vi "Aerotech Controller Module Assembly (main).vi"() -> ()   [LabVIEW 2011]
uses:
  Control 1.ctl
  C:/Users/Admin/Desktop/Gantry Code Transfer/source/Code Transfer/Aerotech.A3200.dll
  Aerotech.A3200.dll
  <vilib>/Utility/error.llb/whitespace.ctl
  <vilib>/Utility/file.llb/Write To Spreadsheet File (DBL).vi
  <vilib>/Utility/file.llb/Write To Spreadsheet File (string).vi
  <vilib>/Utility/file.llb/Read From Spreadsheet File (DBL).vi
panel:
  in  "Load Stored Vectors":bool
  out "Vertical vector":dbl[](array[numeric])
  out "In Range?":bool
  out "Matched?":bool
  out "Match Score":dbl
  out "Station F":bool[](array[boolean])
  out "Station E":bool[](array[boolean])
  in  "Standard Orientation":bool=TRUE
  in  "Station":string
  in  "Module":string
  in  "AlignmentButton":bool
  out "Station A":bool[](array[boolean])
  out "Station B":bool[](array[boolean])
  in  "Stored Vector to Spreadsheet":bool
  out "Encapsulation Pressure":bool
  out "Station D":bool[](array[boolean])
  out "Station C":bool[](array[boolean])
  in  "Storage and Points":enum32{"Stored Vectors", "Index Points"}(tab)
  out "Stored Vectors":T1[][](array[typedef])
  in  "Index Points":string[][](table)
  out "Lock Increment":bool
  in  "Command Array":dbl[][](array[numeric])
  out "Rotation Offset":dbl
  out "Rotate State":bool
  out "Offset":dbl[](array[numeric])
  out "Joystick state":bool
  out "Play/Pause State":bool
  out "Offset State":bool
  out "step stop":bool
  out "goto next state":bool
  out "Current Position":dbl[](array[numeric])=[0.0, -0.0, -0.0, 5.000003999999996] format="%#.3f"
  out "Gantry Head":bool[](array[boolean])
  out "Needle Pressure State":bool
  out "Limit Tripped":bool
  out "Touching":bool
  out "Wait Time":string
  out "Command log":string="\r>"
  in  "Clear Log":bool
  in  "Stop And reset Sequence":bool
  in  "Information":T2(tab)
  in  "Commands":T3(tab)
  in  "Maintenance Position":bool
  in  "Re-Intialize Stored Vectors":bool
  in  "Only Z?":bool
  out "All Axis Mask":i32
  in  "Home button":bool
  in  "Init button":bool
  in  "Axis Indices":u32[](array[ring])=[0, 2, 3, 4] items=["AXIS 1", "AXIS 2", "AXIS 3", "AXIS 4", "AXIS 5", "AXIS 6", "AXIS 7", "AXIS 8", "AXIS 9", "AXIS 10", "AXIS 11", "AXIS 12", "AXIS 13", "AXIS 14", "AXIS 15", "AXIS 16", "AXIS 17", "AXIS 18", "AXIS 19", "AXIS 20", "AXIS 21", "AXIS 22", "AXIS 23", "AXIS 24", "AXIS 25", "AXIS 26", "AXIS 27", "AXIS 28", "AXIS 29", "AXIS 30", "AXIS 31", "AXIS 32"]
  out "CONTROLLER":refnum<k24>
  in  "Autofocus":bool
  in  "Speed":dbl=20.0
  in  "Index Num":dbl
  in  "Index Move":bool
  in  "Angular Speed (deg/s":dbl=2.0
  in  "Use Stored Point?":bool
  in  "Stored Point #":dbl
  in  "Vector Move":bool
  in  "Relative Motion?":bool
  in  "Position (mm)":dbl[](array[numeric])=[0.0, 0.0, 0.0, 0.0]
  in  "Speed (mm/s)":dbl=20.0
  in  "Enable Joystick":bool
  in  "Use Camera?":bool
  in  "Encapsulation Purge":bool
  in  "Set Needle Pressure":bool
  in  "Set Syringe":bool
  in  "Gantry Head Vacuums":bool[](array[boolean])=[FALSE, FALSE, FALSE, FALSE, FALSE, FALSE, FALSE]
  in  "Run Gantry Head Vacuums":bool
  in  "Station Vacuum Controls":enum32{"A", "B", "C", "D", "E", "F"}(tab)
  in  "A \nVacuums":bool[](array[boolean])=[FALSE, FALSE, FALSE, FALSE]
  in  "Run A Vac.":bool
  in  "B Vacuums":bool[](array[boolean])=[FALSE, FALSE, FALSE, FALSE]
  in  "Run B Vac.":bool
  in  "Run C Vacuums":bool
  in  "C Vacuums":bool[](array[boolean])=[FALSE, FALSE, FALSE, FALSE, FALSE, FALSE, FALSE]
  in  "Run D Vacuums":bool
  in  "D Vacuums":bool[](array[boolean])=[FALSE, FALSE, FALSE, FALSE, FALSE, FALSE, FALSE]
  in  "E Vacuums":bool[](array[boolean])=[FALSE, FALSE, FALSE, FALSE, FALSE, FALSE, FALSE]
  in  "Run E Vacuums":bool
  in  "Run F Vacuums":bool
  in  "F Vacuums":bool[](array[boolean])=[FALSE, FALSE, FALSE, FALSE, FALSE, FALSE, FALSE]
  in  "store to":dbl
  in  "point 3":dbl
  in  "point 2":dbl
  in  "point 1":dbl
  in  "center of circle":bool
  in  "Store to":dbl
  in  "Rotate Vector":bool
  in  "Just 3D?":bool
  in  "Store to #'":dbl
  in  "Vector 2":dbl
  in  "Vector 1":dbl
  in  "Calculate Angle":bool
  in  "Store Unit":dbl
  in  "Unitize button":bool
  in  "Unit Vector?":dbl
  in  "Store to Point":dbl
  in  "Scale Vector":bool
  in  "Vector Location":dbl
  in  "Multiplier":dbl
  in  "Store to Vector Pos.":dbl
  in  "Add Vectors":bool
  in  "Add to Vector":dbl
  in  "Vector Addition":dbl[](array[numeric])=[0.0, 0.0, 0.0, 0.0]
  in  "Offset Position":dbl
  in  "Offset from Stored Vector":bool
  in  "Point 1":dbl
  in  "Point 2":dbl
  in  "Store point":dbl
  in  "Distance 2":bool
  in  "Center 2":bool
  in  "Load Index":bool
  in  "Offset Vector":dbl[](array[numeric])=[0.0, 0.0, 0.0, 0.0]
  in  "Set Offset":bool
  in  "Offset Enabled?":bool
  in  "Set Offset State":bool
  in  "Vector to Store":dbl[](array[numeric])=[0.0, 0.0, 0.0, 0.0]
  in  "Store to #":dbl
  in  "Store Vector":bool
  in  "Use Input Vector":bool
  in  "Pt 1":dbl
  in  "Pt 2":dbl
  in  "Store pt":dbl
  in  "Distance":bool
  in  "Center":bool
  in  "Stored point":dbl
  in  "rotation options":dbl
  in  "angle of rotation":dbl
  in  "Wirebond Template":dbl
  in  "Top/Bottom/Left/Right":dbl
  in  "Type of Wire Bond":dbl
  in  "Scan direction T/B":dbl
  in  "Scan direction R/L":dbl
  in  "Wire Bond Finder":bool
  in  "Store rel match to":dbl
  in  "Fiducial Match":bool
  in  "Min Match Score":dbl=600.0
  in  "Move?":bool
  in  "Type of Pat \nMatch":dbl
  in  "Minimum Match Score":sgl=700.0
  out "Faults":string[](array[string])
  in  "Ack Fault":bool
  out "error out":errorcluster
  in  "Command Table":string[][](table)
  in  "Goto Line":bool
  in  "Goto Line Number":dbl
  in  "Load File":bool
  out "Script Details":string
  out "Current Command number":dbl
  in  "Start-Pause":bool
  in  "Step Button":bool
  in  "Zoomtofit":bool
  out "Image":T4(plugin-control)
  out "Image Out":T4(plugin-control)
  in  "movement abort":bool
  in  "EXIT":bool
  # "USE EXIT VI TO STOP PROGRAM PLEASE!"
  # "Y\n\nX\n\nZ\n\nRot"
  # "Right Chuck (HDI)"
  # "Right Chuck (HDI)"
  # "Pickup Head"
  # "Right Chuck (HDI)"
  # "Left Chuck (Module)"
  # "Left Chuck (Module)"
  # "Radial Pickup Head"
  # "Left Chuck (Module)"
  # "Right bridge hold down"
  # "Right bridge hold down"
  # "Center Vacuum"
  # "Right bridge hold down"
  # "Left bridge hold down"
  # "Left bridge hold down"
  # "Left bridge hold down"
  # "Right Chuck (HDI)"
  # "Right Chuck (HDI)"
  # "Right Chuck (HDI)"
  # "Left Chuck (Module)"
  # "Left Chuck (Module)"
  # "Left Chuck (Module)"
  # "Right bridge hold down"
  # "Right bridge hold down"
  # "Right bridge hold down"
  # "Left bridge hold down"
  # "Left bridge hold down"
  # "Left bridge hold down"
  # "0"
  # "1"
  # "2"
  # "3"
  # "4"
  # "5"
  # "6"
  # "7"
  # "8"
  # "9"
  # "10"
  # "Y\n\nX\n\nZ\n\nRot"
  # "Pickup Head"
  # "Radial Pickup Head"
  # "Center Vacuum"
  # "Right Chuck (HDI)"
  # "Left Chuck (Module)"
  # "Right bridge hold down"
  # "Left bridge hold down"
  # "Right Chuck (HDI)"
  # "Left Chuck (Module)"
  # "Right bridge hold down"
  # "Left bridge hold down"
  # "Right Chuck (HDI)"
  # "Left Chuck (Module)"
  # "Right bridge hold down"
  # "Left bridge hold down"
  # "Right Chuck (HDI)"
  # "Left Chuck (Module)"
  # "Right bridge hold down"
  # "Left bridge hold down"
  # "Right Chuck (HDI)"
  # "Left Chuck (Module)"
  # "Right bridge hold down"
  # "Left bridge hold down"
  # "Right Chuck (HDI)"
  # "Left Chuck (Module)"
  # "Right bridge hold down"
  # "Left bridge hold down"
  # "Lateral 2D"
  # "Lateral 3D"
  # "Type of Pattern Match\n0. Nothing\n1. Sensor Fiducial\n2. TR HDI bond pad \n3. TL -----------------\n4. BL -----------------\n5. Simple Edge Scan"
  # "R/L\n0=right to left\n1=left to right\nT/B \n0=top to bottom\n1=bottom to top"
  # "Wire Bond Pattern Matching"
  # "Top/Bottom/Left/Right Pad\n0. Top       2. Left\n1. Bottom  3. Right"
  # "Type of Wire Bond\n0. ROC\n1. HDI\n2. TBM HDI\n3. TBM TOP\n4. Address Bond"
  # "Template\n0. ROC Pad\n1. HDI Pad\n2. RT TBM HDI Pad\n3. RB TBM HDI Pad\n4. BR TBM HDI Pad\n5. BL TBM HDI Pad\n6. LB TBM HDI Pad\n7. LT TBM HDI Pad\n8. TL TBM HDI Pad\n9. TR TBM HDI Pad\n10. TBM TOP TR\n11. TBM TOP BR\n12. TBM TOP BL\n13. TBM TOP TL\n14. Address Bond Top\n15. Address Bond Bottom"
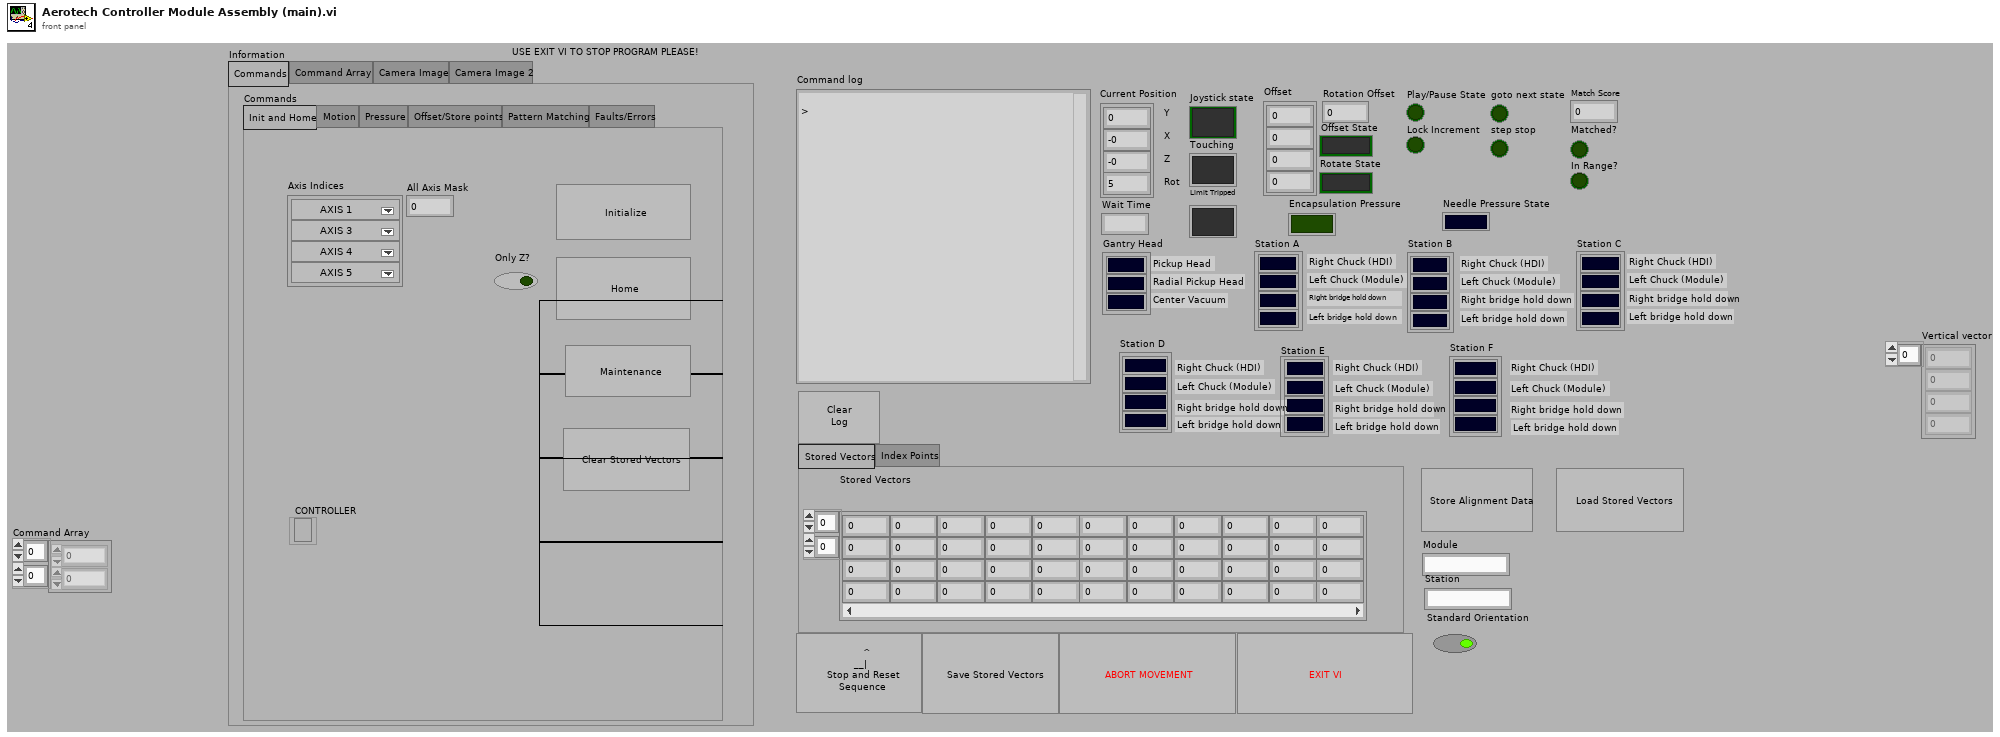
[diagram p1: front panel]
types:
  T1 = typedef "Control 1.ctl" = dbl
  T2 = enum32{"Commands", "Command Array", "Camera Image", "Camera Image 2"}
  T3 = enum32{"Init and Home", "Motion", "Pressure", "Offset/Store points", "Pattern Matching", "Faults/Errors"}
  T4 = typedef "IMAQ Image.ctl" = refnum<image>
  T5 = enum32{"Commands", "Command Array", "Camera Image"}
  T6 = typedef "whitespace.ctl" = u16
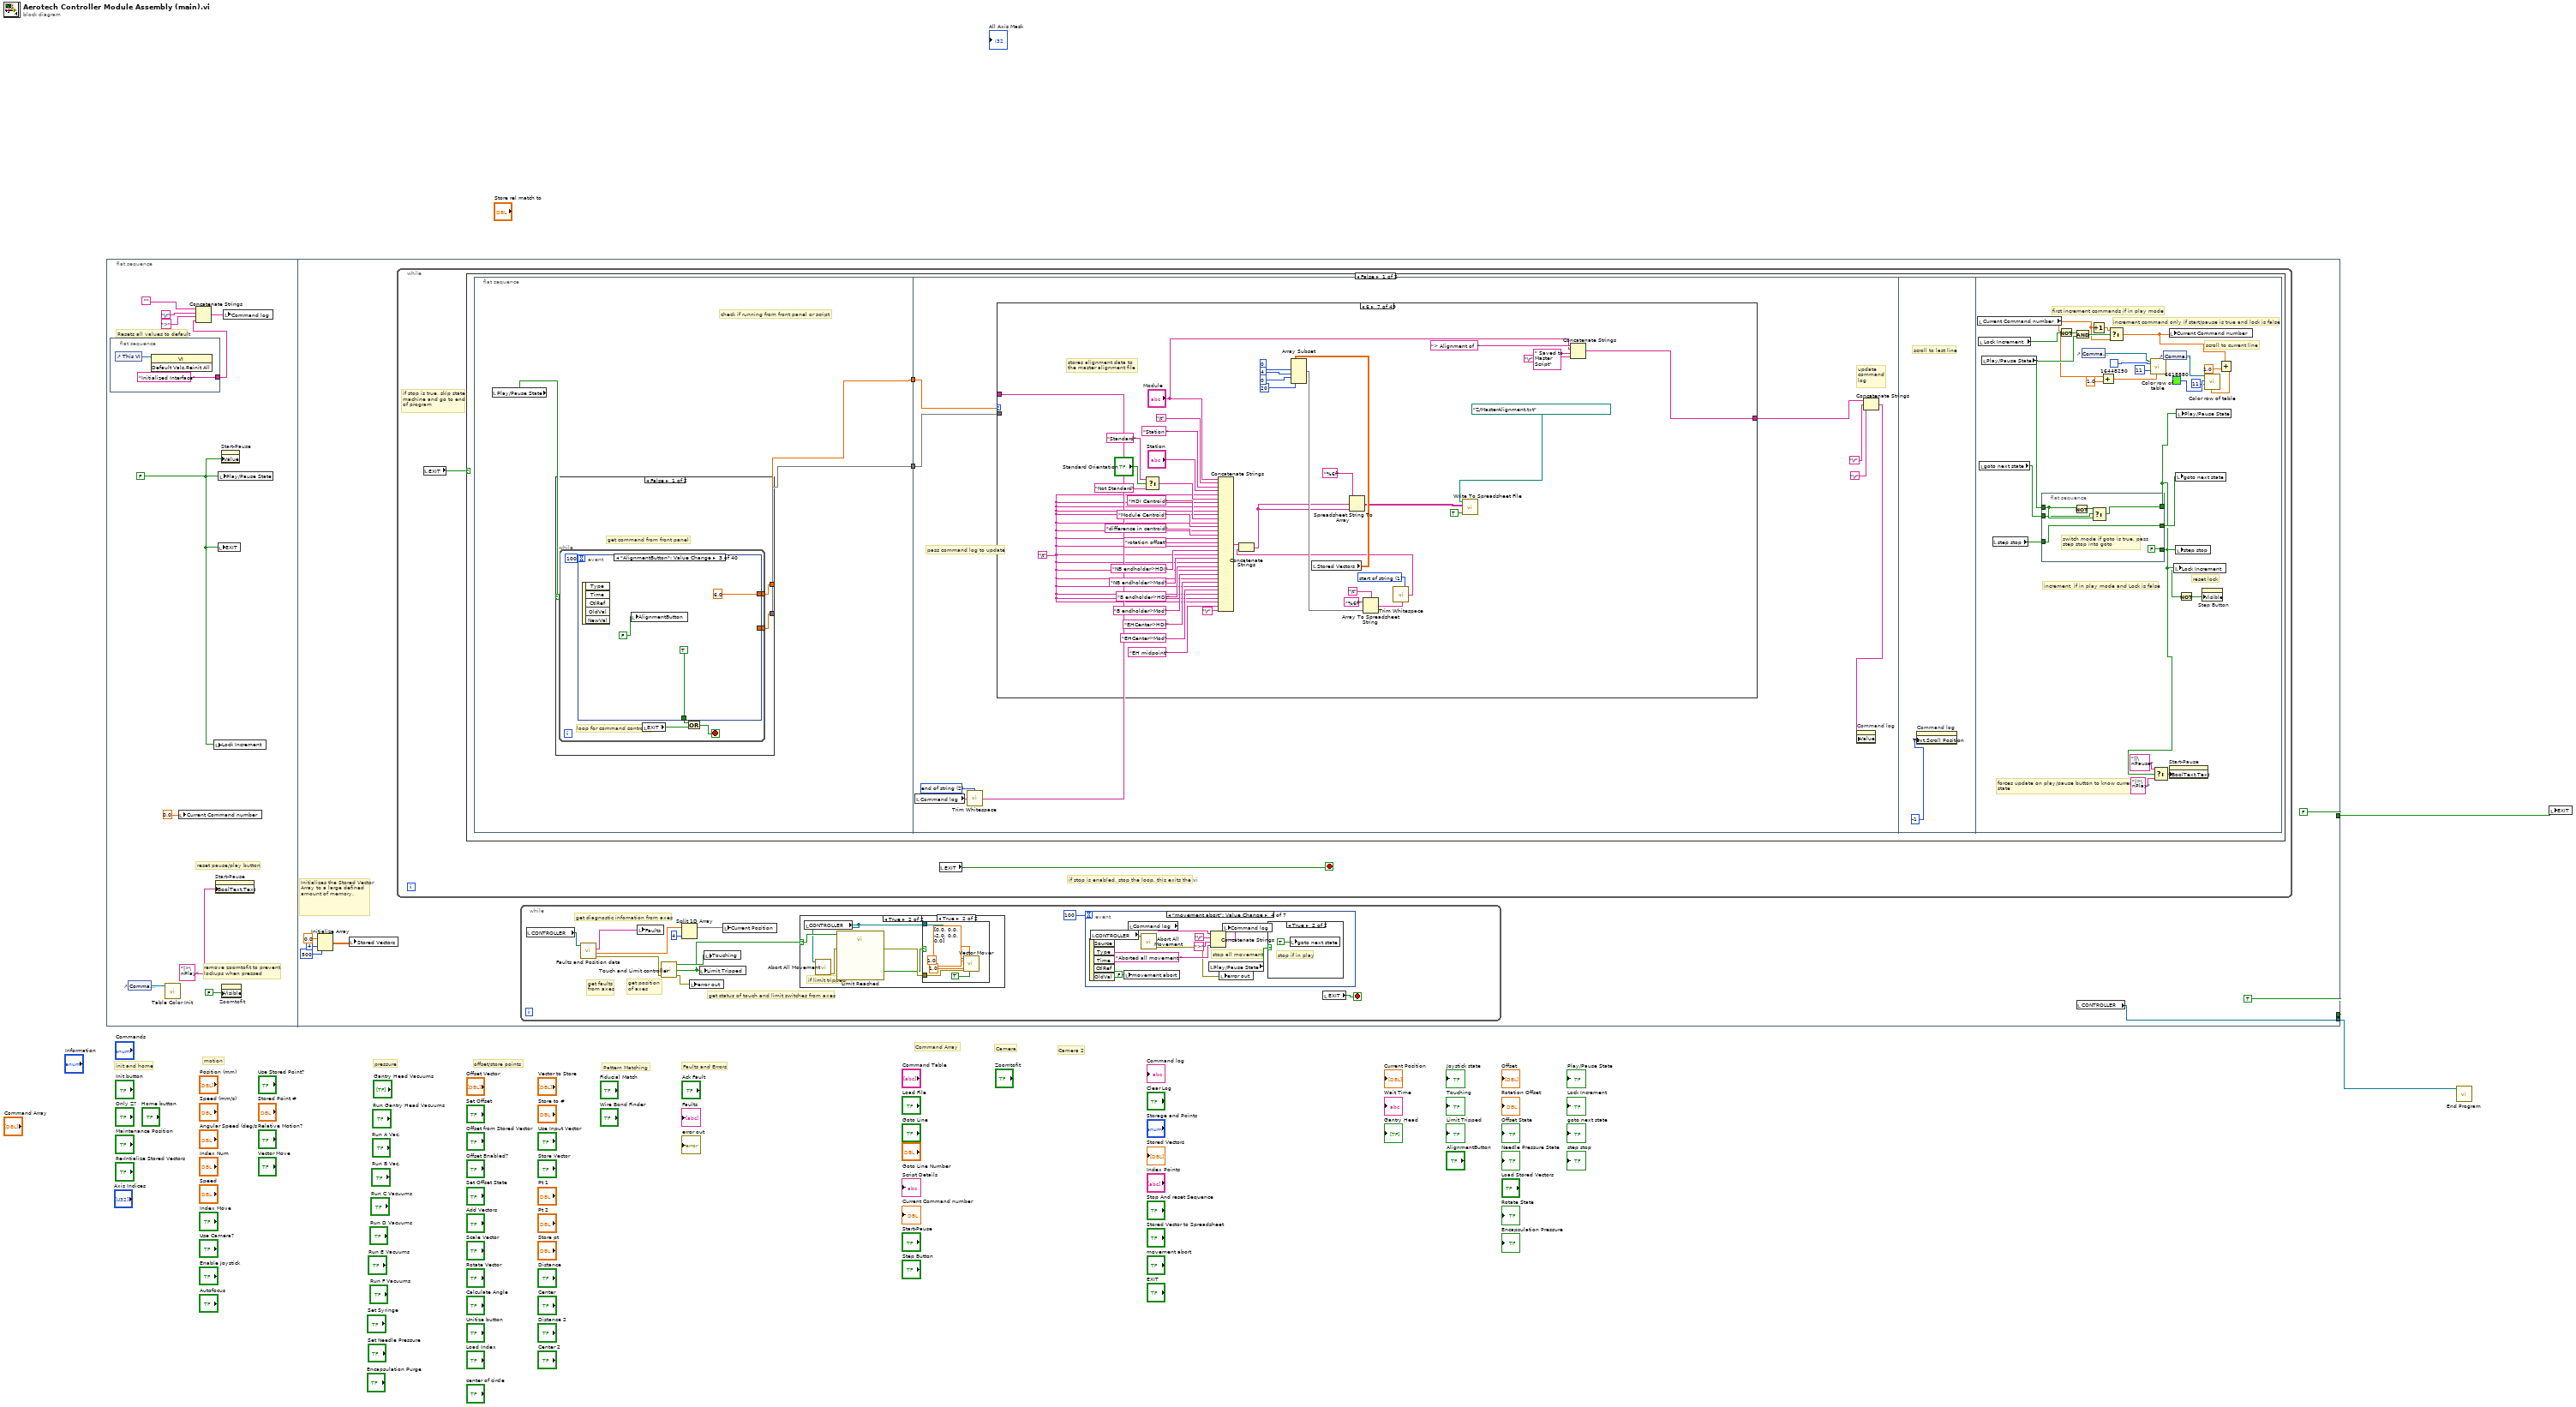
[diagram p0: block diagram]
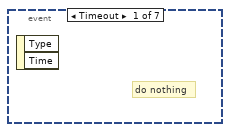
[diagram p4: hidden frame]
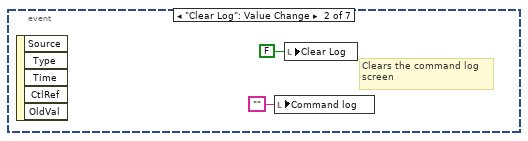
[diagram p5: hidden frame]
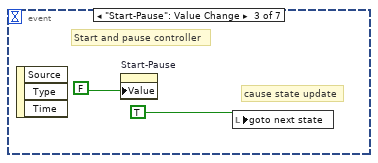
[diagram p6: hidden frame]
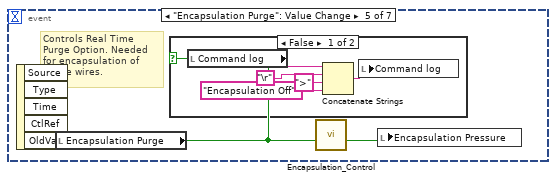
[diagram p8: hidden frame]
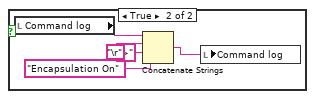
[diagram p9: hidden frame]
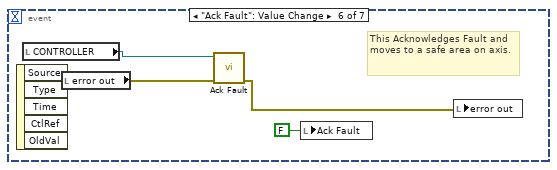
[diagram p10: hidden frame]
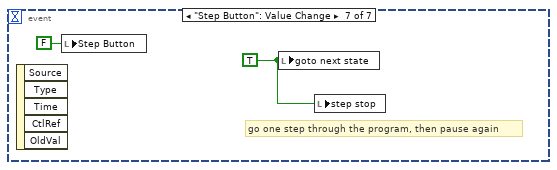
[diagram p11: hidden frame]
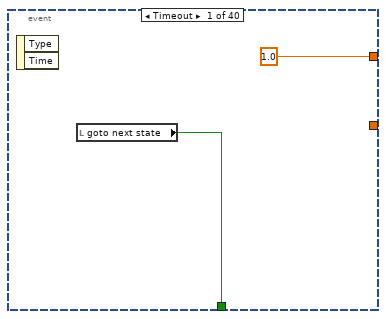
[diagram p12: hidden frame]
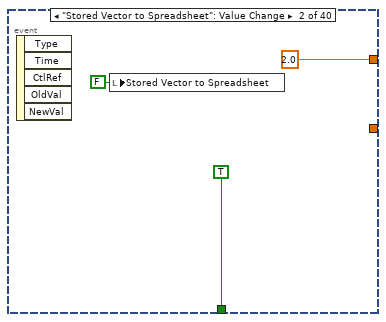
[diagram p13: hidden frame]
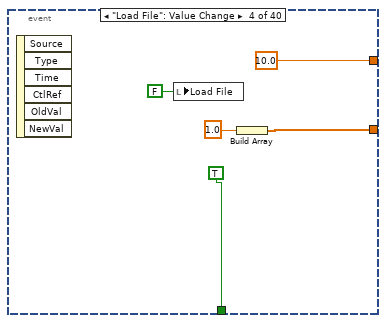
[diagram p14: hidden frame]
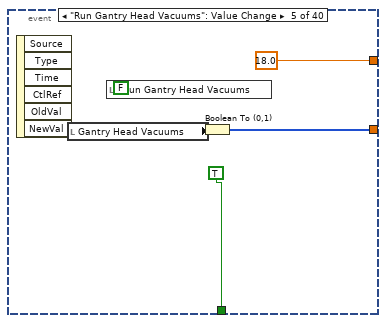
[diagram p15: hidden frame]
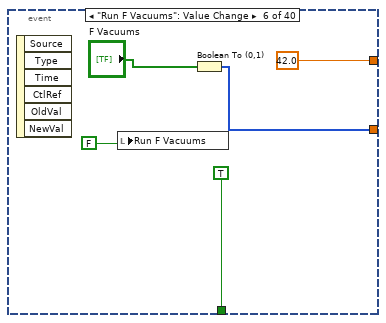
[diagram p16: hidden frame]
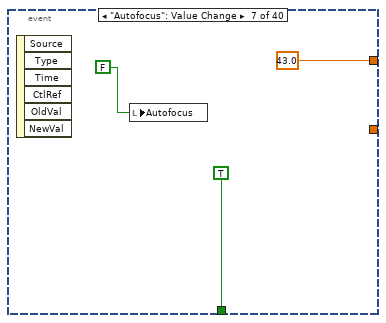
[diagram p17: hidden frame]
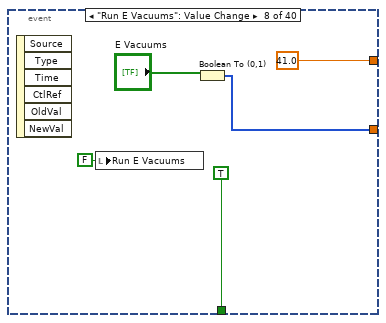
[diagram p18: hidden frame]
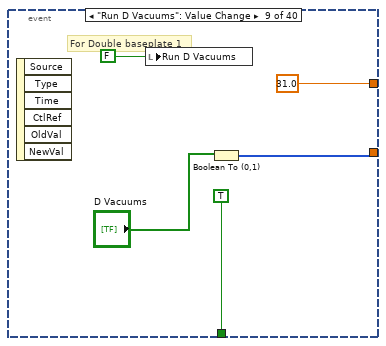
[diagram p19: hidden frame]
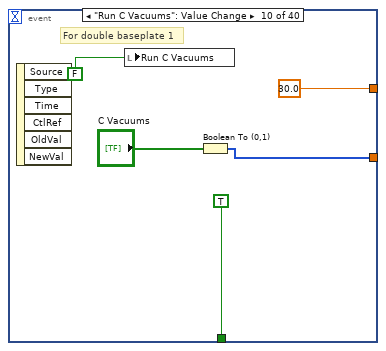
[diagram p20: hidden frame]
diagram:
  # "Camera 2"
  # "Camera"
  # "Command Array"
  # "Faults and Errors"
  # "Pattern Matching"
  # "offset/store points"
  # "pressure"
  # "motion"
  # "init and home"
  n1 = flat-sequence {
    tunnel: [FALSE] -> w2
    tunnel: [w20] -> w1
    tunnel: [TRUE ("All Images? (No)")] -> _
    frame #0 {
      w4 = FALSE ("Start-Pause")
      # "remove zoomtofit to prevent\nlockups when pressed"
      # "reset pause/play button"
      # "Resets all values to default"
      n2 = flat-sequence {
        tunnel: ["Initialized Interface"] -> w6
        frame #0 {
          n3 = control-ref of="This VI"() -> (w14:refnum<vi>)
          n4 = invoke class="VI" method="Default Vals.Reinit All"(reference=w14) -> ()  [unwired: 2 in, 3 out]
        }
      }
      n5 = control-ref of="Command Table"() -> (w3:refnum<vi>)
      n6 = call "Table Color Init.vi"("Table in"=w3) -> ()  [unwired: 11 in]
      n7 = local write "Current Command number"(0.0) -> ()
      n8 = Concatenate Strings("", "\r", ">", w6) -> (w11:string)
      n9 = local write "Lock Increment"(w4) -> ()
      n10 = property on="Start-Pause" class="Bool (strict)"("BoolText.Text"="|>\nPlay" ("Boolean Text.Text")) -> ()  [unwired: 2 in, 2 out]
      n11 = local write "EXIT"(w4) -> ()
      n12 = local write "Play/Pause State"(w4) -> ()
      n13 = property on="Start-Pause" class="Bool (strict)"("Value"=w4) -> ()  [unwired: 2 in, 2 out]
      n14 = property on="Zoomtofit" class="Bool (strict)"("Visible"=FALSE) -> ()  [unwired: 2 in, 2 out]
      n15 = local write "Command log"(w11) -> ()
    }
    frame #1 {
      # "Initializes the Stored Vector Array to a large defined amount of memory."
      n16 = Initialize Array(0.0 ("element"), 4 ("dimension size"), 500 ("dimension size")) -> (w15:dbl[][])
      n17 = local write "Stored Vectors"(w15) -> ()
      n18 = while {
        stop <- w76 stop-if-true
        # "if stop is true, skip state\nmachine and go to end\nof program"
        # "if stop is enabled, stop the loop, this exits the vi"
        n19 = local read "EXIT"() -> (w75:bool)
        n20 = case shown="False" w75 {
          frame False {
            n21 = flat-sequence {
              tunnel: [w79] -> w78
              tunnel: [w81] -> w77
              tunnel: w78 -> [w339]
              tunnel: w77 -> [w338]
              frame #0 {
                # "check if running from front panel or script"
                n22 = local read "Play/Pause State"() -> (w80:bool)
                n23 = case shown="False" w80 {
                  tunnel: [w83 w327] -> w79
                  tunnel: [w82 w326] -> w81
                  frame False {
                    # "get command from front panel"
                    n24 = while {
                      tunnel: [w88] -> w83
                      tunnel: [w87] -> w82
                      stop <- w84 stop-if-true
                      # "loop for command controls"
                      n25 = event shown="[2] \"AlignmentButton\": Value Change" {
                        selector: _ -> [_ _ _ _ _ _ _ _ _ _ _ _ _ _ _ _ _ _ _ _ _ _ _ _ _ _ _ _ _ _ _ _ _ _ _ _ _ _ _ _]
                        dyn-events: _ -> [_ _ _ _ _ _ _ _ _ _ _ _ _ _ _ _ _ _ _ _ _ _ _ _ _ _ _ _ _ _ _ _ _ _ _ _ _ _ _ _]
                        timeout: 100 -> [_ _ _ _ _ _ _ _ _ _ _ _ _ _ _ _ _ _ _ _ _ _ _ _ _ _ _ _ _ _ _ _ _ _ _ _ _ _ _ _]
                        tunnel: [w91 TRUE ("Start/Pause State") TRUE ("Start/Pause State") TRUE ("Start/Pause State") TRUE ("Start/Pause State") TRUE ("Start/Pause State") TRUE ("Start/Pause State") TRUE ("Start/Pause State") TRUE ("Start/Pause State") TRUE ("Start/Pause State") TRUE ("Start/Pause State") TRUE ("Start/Pause State") TRUE ("Start/Pause State") TRUE TRUE ("Start/Pause State") TRUE ("Start/Pause State") TRUE ("Start/Pause State") TRUE ("Start/Pause State") TRUE ("Start/Pause State") TRUE ("Start/Pause State") TRUE ("Start/Pause State") TRUE ("Start/Pause State") TRUE ("Start/Pause State") TRUE ("Start/Pause State") TRUE ("Start/Pause State") TRUE ("Start/Pause State") TRUE ("Start/Pause State") TRUE ("Start/Pause State") TRUE TRUE ("Start/Pause State") TRUE ("Start/Pause State") TRUE ("Start/Pause State") TRUE ("Start/Pause State") TRUE ("Start/Pause State") TRUE ("Start/Pause State") TRUE ("Start/Pause State") TRUE ("Start/Pause State") TRUE ("Start/Pause State") TRUE ("Start/Pause State") TRUE ("Start/Pause State")] -> w86
                        tunnel: [_ _ _ w99 w104 w110 _ w118 w124 w129 w133 w137 w141 w148 w152 w158 _ w163 w174 w187 w195 w197 w208 w217 w220 w225 w233 w238 w244 w252 w258 w273 w278 w284 w291 w295 w306 w315 _ w320] -> w87
                        tunnel: [1.0 ("f") 2.0 ("f") 6.0 ("f") 10.0 ("f") 18.0 ("f") 42.0 ("f") 43.0 ("f") 41.0 ("f") 31.0 ("f") 30.0 ("f") 39.0 ("f") 40.0 ("f") 19.0 ("f") 0.0 ("f") 11.0 ("f") 12.0 ("f") 38.0 ("f") 13.0 ("f") 14.0 ("f") 15.0 ("f") 16.0 ("f") 17.0 ("f") 20.0 ("f") 21.0 ("f") 34.0 ("f") 23.0 ("f") 24.0 ("f") 33.0 ("f") 37.0 ("f") 22.0 ("f") 35.0 ("f") w269 36.0 ("f") 3.0 ("f") 9.0 ("f") 29.0 ("f") 45.0 ("f") 46.0 ("f") 47.0 48.0 ("f")] -> w88
                        event Timeout {
                          n26 = event-data() -> ()  [unwired: 3 out]
                          n27 = local read "goto next state"() -> (w91:bool)
                        }
                        event "Stored Vector to Spreadsheet": Value Change {
                          n28 = event-data() -> ()  [unwired: 6 out]
                          n29 = local write "Stored Vector to Spreadsheet"(FALSE ("Stored Vector to Spreadsheet")) -> ()
                        }
                        event "AlignmentButton": Value Change {
                          n30 = event-data() -> ()  [unwired: 6 out]
                          n31 = local write "AlignmentButton"(FALSE ("AlignmentButton")) -> ()
                        }
                        event "Load File": Value Change {
                          n32 = event-data() -> ()  [unwired: 7 out]
                          n33 = local write "Load File"(FALSE ("Load File")) -> ()
                          n34 = Build Array(1.0 ("C param")) -> (w99:dbl[])
                        }
                        event "Run Gantry Head Vacuums": Value Change {
                          n35 = event-data() -> ()  [unwired: 7 out]
                          n36 = local read "Gantry Head Vacuums"() -> (w105:bool[])
                          n37 = local write "Run Gantry Head Vacuums"(FALSE) -> ()
                          n38 = Boolean To (0,1)(Boolean=w105) -> (0, 1=w104:i16[])
                        }
                        event "Run F Vacuums": Value Change {
                          n39 = event-data() -> ()  [unwired: 7 out]
                          n40 = local write "Run F Vacuums"(FALSE) -> ()
                          n41 = Boolean To (0,1)(Boolean="F Vacuums") -> (0, 1=w110:i16[])
                        }
                        event "Autofocus": Value Change {
                          n42 = event-data() -> ()  [unwired: 7 out]
                          n43 = local write "Autofocus"(FALSE) -> ()
                        }
                        event "Run E Vacuums": Value Change {
                          n44 = event-data() -> ()  [unwired: 7 out]
                          n45 = local write "Run E Vacuums"(FALSE ("Run E Vacuums")) -> ()
                          n46 = Boolean To (0,1)(Boolean="E Vacuums") -> (0, 1=w118:i16[])
                        }
                        event "Run D Vacuums": Value Change {
                          # "For Double baseplate 1"
                          n47 = event-data() -> ()  [unwired: 7 out]
                          n48 = local write "Run D Vacuums"(FALSE ("Run Base Plate 1 Vacuums")) -> ()
                          n49 = Boolean To (0,1)(Boolean="D Vacuums") -> (0, 1=w124:i16[])
                        }
                        event "Run C Vacuums": Value Change {
                          # "For double baseplate 1"
                          n50 = event-data() -> ()  [unwired: 7 out]
                          n51 = local write "Run C Vacuums"(FALSE ("Run Vacuums on New Base Plate")) -> ()
                          n52 = Boolean To (0,1)(Boolean="C Vacuums") -> (0, 1=w129:i16[])
                        }
                        event "Run B Vac.": Value Change {
                          n53 = event-data() -> ()  [unwired: 7 out]
                          n54 = local write "Run B Vac."(FALSE ("Run Right (2) Vac.")) -> ()
                          n55 = Boolean To (0,1)(Boolean="B Vacuums") -> (0, 1=w133:i16[])
                        }
                        event "Run A Vac.": Value Change {
                          n56 = event-data() -> ()  [unwired: 7 out]
                          n57 = local write "Run A Vac."(FALSE ("Run Left (2) Vac.")) -> ()
                          n58 = Boolean To (0,1)(Boolean="A \nVacuums") -> (0, 1=w137:i16[])
                        }
                        event "Set Needle Pressure": Value Change {
                          n59 = event-data() -> ()  [unwired: 7 out]
                          n60 = local read "Set Syringe"() -> (w143:bool)
                          n61 = local write "Set Needle Pressure"(FALSE) -> ()
                          n62 = Boolean To (0,1)(Boolean=w143) -> (0, 1=w142:i16)
                          n63 = Build Array(w142) -> (w141:i16[])
                        }
                        event "Stop And reset Sequence": Value Change {
                          n64 = event-data() -> ()  [unwired: 7 out]
                          n65 = local write "Stop And reset Sequence"(FALSE ("Stop And reset Sequence")) -> ()
                          n66 = Build Array(0.0 ("C param")) -> (w148:dbl[])
                        }
                        event "Load Stored Vectors": Value Change {
                          n67 = event-data() -> ()  [unwired: 7 out]
                          n68 = Build Array(0.0 ("C param")) -> (w152:dbl[])
                        }
                        event "Init button": Value Change {
                          n69 = event-data() -> ()  [unwired: 7 out]
                          n70 = local read "Axis Indices"() -> (w158:u32[])
                          n71 = local write "Init button"(FALSE ("Init button")) -> ()
                        }
                        event "Re-Intialize Stored Vectors": Value Change {
                          n72 = event-data() -> ()  [unwired: 7 out]
                          n73 = local write "Re-Intialize Stored Vectors"(FALSE ("Re-Intialize Stored Vectors")) -> ()
                        }
                        event "Home button": Value Change {
                          n74 = event-data() -> ()  [unwired: 7 out]
                          n75 = local read "Only Z?"() -> (w165:bool)
                          n76 = local write "Home button"(FALSE ("Home button")) -> ()
                          n77 = Boolean To (0,1)(Boolean=w165) -> (0, 1=w164:i16)
                          n78 = Build Array(w164) -> (w163:i16[])
                        }
                        event "Vector Move": Value Change {
                          n79 = event-data() -> ()  [unwired: 7 out]
                          n80 = local read "Relative Motion?"() -> (w175:bool)
                          n81 = local read "Speed (mm/s)"() -> (w169:dbl)
                          n82 = local read "Use Stored Point?"() -> (w171:bool)
                          n83 = case shown="True" w171 {
                            tunnel: [w180 w186] -> w170
                            frame False {
                              n84 = local read "Position (mm)"() -> (w182:dbl[])
                              n85 = Build Array (concatenate)(0, w182) -> (w180:dbl[])
                            }
                            frame True {
                              w183 = 0.0 ("element")
                              n86 = local read "Stored Point #"() -> (w184:dbl)
                              n87 = Build Array(1.0 ("element"), w184, w183, w183, w183) -> (w186:dbl[])
                            }
                          }
                          n88 = Select(t=1.0, s=w175, f=0.0) -> (s? t:f=w173:dbl)
                          n89 = local write "Vector Move"(FALSE ("Vector Move")) -> ()
                          n90 = Build Array (concatenate)(w170, w169, w173) -> (w174:dbl[])
                        }
                        event "Enable Joystick": Value Change {
                          n91 = event-data() -> ()  [unwired: 7 out]
                          n92 = local read "Use Camera?"() -> (w189:bool)
                          n93 = Boolean To (0,1)(Boolean=w189) -> (0, 1=w188:i16)
                          n94 = local write "Enable Joystick"(FALSE) -> ()
                          n95 = Build Array(w188) -> (w187:i16[])
                        }
                        event "Set Offset": Value Change {
                          n96 = event-data() -> ()  [unwired: 7 out]
                          n97 = local read "Offset Vector"() -> (w195:dbl[])
                          n98 = local write "Set Offset"(FALSE ("Set Offset")) -> ()
                        }
                        event "Goto Line": Value Change {
                          n99 = event-data() -> ()  [unwired: 7 out]
                          n100 = local read "Goto Line Number"() -> (w198:dbl)
                          n101 = local write "Goto Line"(FALSE ("Goto Line")) -> ()
                          n102 = Build Array(w198) -> (w197:dbl[])
                        }
                        event "Store Vector": Value Change {
                          n103 = event-data() -> ()  [unwired: 7 out]
                          n104 = local read "Use Input Vector"() -> (w206:bool)
                          n105 = local read "Vector to Store"() -> (w203:dbl[])
                          n106 = local read "Store to #"() -> (w210:dbl)
                          n107 = local write "Store Vector"(FALSE ("Store Point")) -> ()
                          n108 = Not(x="Just 3D?") -> (.not. x?=w205:bool)
                          n109 = Boolean To (0,1)(Boolean=w205) -> (0, 1=w202:i16)
                          n110 = Not(x=w206) -> (.not. x?=w207:bool)
                          n111 = Boolean To (0,1)(Boolean=w207) -> (0, 1=w209:i16)
                          n112 = Build Array (concatenate)(w210, w209, w203, w202) -> (w208:dbl[])
                        }
                        event "Set Offset State": Value Change {
                          n113 = event-data() -> ()  [unwired: 7 out]
                          n114 = local read "Offset Enabled?"() -> (w216:bool)
                          n115 = local write "Set Offset State"(FALSE ("Set Offset State")) -> ()
                          n116 = Boolean To (0,1)(Boolean=w216) -> (0, 1=w218:i16)
                          n117 = Build Array(w218) -> (w217:i16[])
                        }
                        event "Offset from Stored Vector": Value Change {
                          n118 = event-data() -> ()  [unwired: 7 out]
                          n119 = Build Array("Offset Position") -> (w220:dbl[])
                        }
                        event "Distance": Value Change {
                          n120 = event-data() -> ()  [unwired: 7 out]
                          n121 = local read "Store pt"() -> (w226:dbl)
                          n122 = local read "Pt 2"() -> (w227:dbl)
                          n123 = local read "Pt 1"() -> (w228:dbl)
                          n124 = local write "Distance"(FALSE ("Distance")) -> ()
                          n125 = Build Array(w228, w227, w226) -> (w225:dbl[])
                        }
                        event "Calculate Angle": Value Change {
                          n126 = event-data() -> ()  [unwired: 7 out]
                          n127 = Build Array("Vector 1", "Vector 2", "Store to #'") -> (w233:dbl[])
                        }
                        event "Distance 2": Value Change {
                          n128 = event-data() -> ()  [unwired: 7 out]
                          n129 = local write "Distance 2"(FALSE ("Distance 2")) -> ()
                          n130 = Build Array("Point 1", "Point 2", "Store point") -> (w238:dbl[])
                        }
                        event "Center 2": Value Change {
                          n131 = event-data() -> ()  [unwired: 7 out]
                          n132 = local write "Center 2"(FALSE ("Center 2")) -> ()
                          n133 = local read "Store point"() -> (w247:dbl)
                          n134 = local read "Point 1"() -> (w245:dbl)
                          n135 = local read "Point 2"() -> (w246:dbl)
                          n136 = Build Array(w245, w246, w247) -> (w244:dbl[])
                        }
                        event "Center": Value Change {
                          n137 = event-data() -> ()  [unwired: 7 out]
                          n138 = local read "Store pt"() -> (w251:dbl)
                          n139 = local read "Pt 1"() -> (w254:dbl)
                          n140 = local read "Pt 2"() -> (w253:dbl)
                          n141 = Build Array(w254, w253, w251) -> (w252:dbl[])
                          n142 = local write "Center"(FALSE ("Center")) -> ()
                        }
                        event "Add Vectors": Value Change {
                          n143 = event-data() -> ()  [unwired: 7 out]
                          n144 = local write "Add Vectors"(FALSE ("Add Vectors")) -> ()
                          n145 = Build Array (concatenate)("Vector Addition", "Add to Vector", "Store to Vector Pos.") -> (w258:dbl[])
                        }
                        event "Fiducial Match": Value Change {
                          n146 = event-data() -> ()  [unwired: 7 out]
                          n147 = local write "Fiducial Match"(FALSE) -> ()
                          n148 = local read "Store rel match to"() -> (w272:dbl)
                          n149 = case shown="True" "Move?" {
                            tunnel: [28.0 ("f") 44.0 ("f")] -> w269
                            frame False {
                            }
                            frame True {
                            }
                          }
                          n150 = Build Array("Type of Pat \nMatch", w272, "Min Match Score", "Scan direction R/L", "Scan direction T/B") -> (w273:dbl[])
                        }
                        event "Scale Vector": Value Change {
                          n151 = event-data() -> ()  [unwired: 7 out]
                          n152 = local write "Scale Vector"(FALSE ("Scale Vector")) -> ()
                          n153 = Build Array("Multiplier", "Vector Location", "Store to Point") -> (w278:dbl[])
                        }
                        event "Unitize button": Value Change {
                          n154 = event-data() -> ()  [unwired: 7 out]
                          n155 = local write "Unitize button"(FALSE ("Unitize button")) -> ()
                          n156 = Build Array("Unit Vector?", "Store Unit") -> (w284:dbl[])
                        }
                        event "Load Index": Value Change {
                          n157 = event-data() -> ()  [unwired: 7 out]
                          n158 = local write "Load Index"(FALSE ("Load Index")) -> ()
                          n159 = Build Array(1) -> (w291:i32[])
                        }
                        event "Index Move": Value Change {
                          n160 = event-data() -> ()  [unwired: 7 out]
                          n161 = local write "Index Move"(FALSE ("Index Move")) -> ()
                          n162 = local read "Index Num"() -> (w298:dbl)
                          n163 = local read "Speed"() -> (w296:dbl)
                          n164 = Build Array(w298, w296) -> (w295:dbl[])
                        }
                        event "Wire Bond Finder": Value Change {
                          n165 = event-data() -> ()  [unwired: 7 out]
                          n166 = local write "Wire Bond Finder"(FALSE ("ROC Finder")) -> ()
                          n167 = Build Array("Type of Wire Bond", "Minimum Match Score", "Top/Bottom/Left/Right", "Wirebond Template") -> (w306:dbl[])
                        }
                        event "Rotate Vector": Value Change {
                          n168 = event-data() -> ()  [unwired: 7 out]
                          n169 = local write "Rotate Vector"(FALSE ("Rotate Vector")) -> ()
                          n170 = Build Array("Stored point", "Store to", "rotation options", "angle of rotation") -> (w315:dbl[])
                        }
                        event "Maintenance Position": Value Change {
                          n171 = event-data() -> ()  [unwired: 7 out]
                        }
                        event "center of circle": Value Change {
                          n172 = event-data() -> ()  [unwired: 7 out]
                          n173 = Build Array("point 1", "point 2", "point 3", "store to") -> (w320:dbl[])
                        }
                      }
                      n174 = local read "EXIT"() -> (w85:bool)
                      n175 = Or(x=w86, y=w85) -> (x .or. y?=w84:bool)
                    }
                  }
                  frame True {
                    # "Command \nand param"
                    # "make the cursor slightly different to notice\nwhether in step or play"
                    # "script control\ngrabs command\nfrom command\narray"
                    # "running from script, no parameters will be passed from \nfront panel."
                    n176 = local read "Current Command number"() -> (w329:dbl)
                    n177 = local read "Command Array"() -> (w328:dbl[][])
                    n178 = Index Array(array=w328, index (row)=w329) -> (element=w330:dbl[])  [unwired: 1 in]
                    n179 = Split 1D Array(array=w330, index=1) -> (first subarray=w333:dbl[], second subarray=w326:dbl[])
                    n180 = Index Array(array=w333, index=0) -> (element=w327:dbl)
                  }
                }
              }
              frame #1 {
                w336 = T6 2 items=["both", "start of string", "end of string"] ("location (both)")
                # "pass command log to update"
                # "update\ncommand\nlog"
                n181 = local read "Command log"() -> (w337:string)
                n182 = call <vilib>:"Trim Whitespace.vi"("string"=w337, "location (both)"=w336) -> ("trimmed string"=w335:string)
                n183 = case shown="6" w339 {
                  tunnel: w338 -> [_ _ _ w401 w411 w434 _ _ _ w518 w542 _ _ w583 w599 w647 w696 w710 w732 w748 w755 w803 w831 w852 w884 _ w904 w918 w929 w965 w971 w992 w1011 w1040 w1043 w1069 w1095 w1108 _ w1135 w1154 w1174 w1192 _ w1216 w1330 w1456 _ w1516]
                  tunnel: w335 -> [w345 w361 w369 w402 w412 w437 _ w495 w508 w523 w536 w559 w571 w587 w614 w654 w702 w712 w734 w750 w770 w805 w835 w855 w873 w892 w906 w920 w942 w950 w972 w991 w1007 w1022 w1047 w1076 w1099 w1109 w1125 w1136 w1155 w1175 w1194 w1212 w1220 w1334 w1428 w1481 w1492]
                  tunnel: [w344 w361 w367 w383 w407 w436 w482 w494 w507 w522 w535 w558 w570 w584 w605 w648 w701 w711 w733 w749 w769 w804 w834 w854 w872 w891 w905 w919 w935 w946 w970 w990 w1008 w1021 w1046 w1075 w1096 w1100 w1124 w1133 w1152 w1172 w1193 w1211 w1219 w1333 w1427 w1480 w1491] -> w334
                  frame 0, Default {
                    # "This prevents the command from \nincrementing when pressing the stop and\nreset key."
                    # "Stop and reset command, used to end script as well"
                    n184 = local read "Play/Pause State"() -> (w352:bool)
                    n185 = local read "EXIT"() -> (w351:bool)
                    n186 = case shown="True" w352 {
                      tunnel: [w356 "End Program "] -> w347
                      tunnel: w351 -> [w357 _]
                      frame False {
                        n187 = local write "goto next state"(FALSE ("stop")) -> ()
                        n188 = Select(t="", s=w357, f="Reset ") -> (s? t:f=w356:string)
                      }
                      frame True {
                        n189 = local write "goto next state"(TRUE) -> ()
                      }
                    }
                    n190 = control-ref of="Command Table"() -> (w343:refnum<vi>)
                    n191 = Build Array("\r", ">", w347) -> (w346:string[])
                    n192 = local write "Current Command number"(0.0 ("Current Command number")) -> ()
                    n193 = call "Table Color Init.vi"("Table in"=w343) -> ()  [unwired: 11 in]
                    n194 = call "String array concatenation.vi"("Array of Strings"=w346, "Input String"=w345) -> ("Concatenated Array"=w344:string)  [unwired: 2 in]
                    n195 = local write "Lock Increment"(TRUE) -> ()
                  }
                  frame 1 {
                    # "comment line command"
                    # "does nothing, makes file reading easier with padding"
                  }
                  frame 2 {
                    # "Store Vectors"
                    n196 = local read "Stored Vectors"() -> (w370:T1[][])
                    n197 = call "File Dialog"("default name"="Stored Vectors") -> ("selected path"=w364:path, "error out"=w362:errorcluster)  [unwired: 11 in, 2 out]
                    n198 = case shown="No Error" w362 {
                      tunnel: w370 -> [w374 _]
                      tunnel: [w372 "Save Stored Vectors Cancelled"] -> w365
                      tunnel: w364 -> [w371 _]
                      frame No Error {
                        n199 = call-poly <vilib>:"Write To Spreadsheet File.vi"("2D data"=w374, "file path (dialog if empty)"=w371) -> ("new file path (Not A Path if cancelled)"=w373:path)  [unwired: 6 in]
                        n200 = Path To String(path=w373) -> (string=w372:string)
                      }
                      frame Error {
                      }
                    }
                    n201 = Concatenate Strings(w369, "> Stored Vectors Output to :" ("string"), "\r", w365) -> (w367:string)
                  }
                  frame 3 {
                    # "Will ignore rotation, we want a 3D unit vector not 4D."
                    # "Will return a unit vector of a selected vector in the Stored Vectors array."
                    n202 = Index Array(array=w401) -> (element #1=w388:dbl, element #2=w385:dbl)  [unwired: 2 in]
                    n203 = local read "Stored Vectors"() -> (w400:T1[][])
                    n204 = Index Array(array=w400, index (col)=w388) -> (element=w382:T1[])  [unwired: 1 in]
                    n205 = Number To Decimal String(number=w388) -> (decimal integer string=w387:string)  [unwired: 1 in]
                    n206 = Index Array(array=w382) -> (element #1=w399:T1, element #2=w398:T1, element #3=w397:T1)  [unwired: 3 in]
                    n207 = Number To Decimal String(number=w385) -> (decimal integer string=w384:string)  [unwired: 1 in]
                    n208 = Square(x=w399) -> (x^2=w394:T1)
                    n209 = Square(x=w398) -> (x^2=w395:T1)
                    n210 = Square(x=w397) -> (x^2=w396:T1)
                    n211 = Replace Array Subset(array=w382, new element=T1 0.0 ("new element/subarray"), index=3) -> (w379:T1[])
                    n212 = Build Array(w394, w395, w396) -> (w393:T1[])
                    n213 = Add Array Elements(numeric array=w393) -> (sum=w377:T1)
                    n214 = Concatenate Strings(w402, "\r", ">Unit Vector of slot " ("string"), w387, "     Stored to :" ("string"), w384) -> (w383:string)
                    n215 = Square Root(x=w377) -> (sqrt(x)=w376:T1)
                    n216 = Divide(x=w379, y=w376) -> (x/y=w378:T1[])
                    n217 = local read "Stored Vectors"() -> (w392:T1[][])
                    n218 = Replace Array Subset(array=w392, new element=w378, index (col)=w385) -> (w391:T1[][])  [unwired: 1 in]
                    n219 = local write "Stored Vectors"(w391) -> ()
                  }
                  frame 4 {
                    # "seconds"
                    # "minutes"
                    n220 = Index Array(array=w411, index #1=0 ("index"), index #2=1 ("index")) -> (element #1=w409:dbl, element #2=w403:dbl)
                    n221 = Multiply(x=60.0, y=w409) -> (x*y=w405:dbl)
                    n222 = Add(x=w405, y=w403) -> (x+y=w404:dbl)
                    n223 = while {
                      shift-right: [w418] -> _
                      shift-left: w404 -> [w416]
                      stop <- w426 stop-if-true
                      w421 = i16 2 ("width (-)")
                      n224 = Wait (ms)(milliseconds to wait=u32 10) -> ()  [unwired: 1 out]
                      n225 = Quotient & Remainder(x=w416, y=60.0) -> (x-y*floor(x/y)=w423:dbl, floor(x/y)=w422:dbl)
                      n226 = Number To Decimal String(number=w423, width (-)=w421) -> (decimal integer string=w419:string)
                      n227 = Number To Decimal String(number=w422, width (-)=w421) -> (decimal integer string=w420:string)
                      n228 = Concatenate Strings(w420, ":", w419) -> (w424:string)
                      n229 = Less Or Equal?(x=w416, y=0.0) -> (x <= y?=w426:bool)
                      n230 = local write "Wait Time"(w424) -> ()
                      n231 = Subtract(x=w416, y=0.01) -> (x-y=w418:dbl)
                    }
                    n232 = Concatenate Strings(w412, "\r", ">", "Waiting ") -> (w407:string)
                    n233 = local write "Command log"(w407) -> ()
                  }
                  frame 5 {
                    # "This pauses execution and goes into free form mode, also forces command number up by one since next frame will not."
                    n234 = Array To Spreadsheet String(delimiter (Tab)=",", array=w434, 3:"") -> (spreadsheet string=w431:string)
                    n235 = property on="Start-Pause" class="Bool (strict)"("Val(Sgnl)"=FALSE ("Value (Signaling)")) -> ()  [unwired: 2 in, 2 out]
                    n236 = local write "goto next state"(TRUE ("goto next state")) -> ()
                    n237 = Concatenate Strings(w437, "\r", ">", "Paused ", w431) -> (w436:string)
                  }
                  frame 6 {
                    w441 = "\t" ("string")
                    w461 = T6 1 items=["both", "start of string", "end of string"] ("location (both)")
                    # "stores alignment data to the master alignment file"
                    n238 = Select(t="Standard", s="Standard Orientation", f="Not Standard") -> (s? t:f=w455:string)
                    n239 = Concatenate Strings("Module", "\t" ("string"), "Station " ("string"), "Station", w441, w455, w441, w441, w441, w441, "HDI Centroid" ("string"), w441, "Module Centroid" ("string"), w441, "difference in centroid" ("string"), w441, "rotation offset" ("string"), w441, "NB endholder>HDI" ("string"), w441, "NB endholder>Mod" ("string"), w441, "B endholder>HDI" ("string"), w441, "B endholder>Mod" ("string"), w441, "EHCenter>HDI" ("string"), w441, "EHCenter>Mod" ("string"), w441, w441, w441, "EH midpoint" ("string"), "\r") -> (w464:string)
                    n240 = local read "Stored Vectors"() -> (w471:T1[][])
                    n241 = Array Subset(array=w471, index (row)=0 ("index"), length (row)=4 ("length"), index (col)=0 ("length"), length (col)=20 ("length")) -> (w470:T1[][])
                    n242 = Array To Spreadsheet String(delimiter (Tab)="\t" ("string"), array=w470, 3:"%6f" ("format string")) -> (spreadsheet string=w463:string)
                    n243 = call <vilib>:"Trim Whitespace.vi"("string"=w463, "location (both)"=w461) -> ("trimmed string"=w462:string)
                    n244 = Concatenate Strings(w464, w462) -> (w460:string)
                    n245 = Spreadsheet String To Array(format string="%6f", spreadsheet string=w460, array type (2D Dbl)=w460) -> (array=w458:string[][])  [unwired: 1 in]
                    n246 = call-poly <vilib>:"Write To Spreadsheet File.vi"("append to file? (new file:F)"=TRUE, "2D data"=w458, "file path (dialog if empty)"=path "Z:/MasterAlignment.txt") -> ()  [unwired: 5 in, 1 out]
                    n247 = Concatenate Strings("> Alignment of  " ("string"), "Module", " Saved to Master Script" ("string"), "\r") -> (w482:string)
                  }
                  frame 7 {
                    w491 = T1[] [64.322, 0.419, 0.0, 0.0] ("new element/subarray")
                    w485 = 8 ("disabled index (col)")
                    # "Stamp Vector Taken from the \nCalibration File in the path:\n:\\Documents and Settings\\local-admin\\Desktop\\Main_Module_Assembly"
                    # "Stores the rotation vector for the stamp in the stored vectors array"
                    n248 = local read "Stored Vectors"() -> (w493:T1[][])
                    n249 = Replace Array Subset(array=w493, new element=w491, index (col)=w485) -> (w492:T1[][])  [unwired: 1 in]
                    n250 = Number To Decimal String(number=w485) -> (decimal integer string=w484:string)  [unwired: 1 in]
                    n251 = Array To Spreadsheet String(delimiter (Tab)=", ", array=w491, 3:"%6f" ("format string")) -> (spreadsheet string=w487:string)
                    n252 = Concatenate Strings(w495, "\r", ">", "Rotation Vector for Stamp:  " ("string"), "\r", w487, "Stored to: " ("string"), w484) -> (w494:string)
                    n253 = local write "Stored Vectors"(w492) -> ()
                  }
                  frame 8 {
                    w504 = dbl[] [0.673, -0.309, 0.0, 0.0, 0.0] ("Movement Vector")
                    n254 = local read "Angular Speed (deg/s"() -> (w500:dbl)
                    n255 = local read "CONTROLLER"() -> (w499:refnum<k24>)
                    n256 = call "Vector Mover.vi"("Absolute/Relative (F/T)"=TRUE, "Movement Vector"=w504, "Angular Speed"=w500, "Vector Speed"=1.0, "controller in"=w499) -> ("error out"=w498:errorcluster)  [unwired: 3 in, 1 out]
                    n257 = Array To Spreadsheet String(delimiter (Tab)=", ", array=w504, 3:"%6f" ("format string")) -> (spreadsheet string=w502:string)
                    n258 = Concatenate Strings(w508, "\r", ">", "Stamp Centered by amount:  " ("string"), "\r", w502) -> (w507:string)
                    n259 = local write "error out"(w498) -> ()
                  }
                  frame 9 {
                    # "Load an Index File"
                    n260 = Current VI's Path() -> (path=w515:path)
                    n261 = Index Array(array=w518, index=0) -> (element=w520:dbl)
                    n262 = Equal?(x=w520, y=1.0) -> (x = y?=w517:bool)
                    n263 = Build Path(base path=w515, name or relative path="Index.csv") -> (appended path=w513:path)
                    n264 = case shown="True" w517 {
                      tunnel: ["Index Load Failed" "Index Loaded"] -> w516
                      tunnel: w513 -> [_ _]
                      frame False {
                      }
                      frame True {
                        n265 = call "Open Index File.vi"() -> ("Array of points"=w529:string[][])  [unwired: 11 in]
                        n266 = local write "Index Points"(w529) -> ()
                      }
                    }
                    n267 = Build Array("\r", ">", w516) -> (w524:string[])
                    n268 = call "String array concatenation.vi"("Array of Strings"=w524, "Input String"=w523) -> ("Concatenated Array"=w522:string)  [unwired: 2 in]
                  }
                  frame 10 {
                    # "reset command number"
                    # "This is the load file case"
                    n269 = control-ref of="Command Table"() -> (w530:refnum<vi>)
                    n270 = Index Array(array=w542, index=0) -> (element=w540:dbl)
                    n271 = Equal?(x=w540, y=1.0) -> (x = y?=w538:bool)
                    n272 = call "Table Color Init.vi"("Table in"=w530) -> ()  [unwired: 11 in]
                    n273 = local write "Current Command number"(0.0 ("Current Command number")) -> ()
                    n274 = case shown="True" w538 {
                      tunnel: ["Wrong parameters to load file" w548] -> w532
                      frame False {
                      }
                      frame True {
                        # "opens file and outputs\nin table and array form"
                        # "This loads a file into the  command array for later use, files in CSV format"
                        n275 = call "Open file in table.vi"() -> ("Error Out"=w547:errorcluster, "Command Array"=w545:dbl[][], "Command Table"=w546:string[][], "Details"=w544:string)  [unwired: 7 in, 1 out]
                        n276 = case shown="No Error" w547 {
                          tunnel: ["File Loaded " "File Load Cancelled "] -> w548
                          tunnel: w546 -> [w551 _]
                          tunnel: w545 -> [w550 _]
                          tunnel: w544 -> [w549 _]
                          frame No Error {
                            # "Only if not cancelled will file load"
                            n277 = local write "Script Details"(w549) -> ()
                            n278 = local write "Command Table"(w551) -> ()
                            n279 = local write "Command Array"(w550) -> ()
                          }
                          frame Error {
                          }
                        }
                      }
                    }
                    n280 = Build Array("\r", ">", w532) -> (w537:string[])
                    n281 = call "String array concatenation.vi"("Array of Strings"=w537, "Input String"=w536) -> ("Concatenated Array"=w535:string)  [unwired: 2 in]
                  }
                  frame 11 {
                    n282 = call "File Dialog2"("default name"="Stored Vectors") -> ("selected path"=w557:path, "error out"=w555:errorcluster)  [unwired: 11 in, 2 out]
                    n283 = case shown="No Error" w555 {
                      tunnel: w557 -> [w565 _]
                      tunnel: ["Success!" "Save Stored Vectors Cancelled"] -> w554
                      frame No Error {
                        n284 = call-poly <vilib>:"Read From Spreadsheet File.vi"("file path (dialog if empty)"=w565) -> ("all rows"=w564:dbl[][])  [unwired: 6 in, 4 out]
                        n285 = local write "Stored Vectors"(w564) -> ()
                      }
                      frame Error {
                      }
                    }
                    n286 = Concatenate Strings(w559, "\r", ">", "Stored Vectors Loaded ", w554) -> (w558:string)
                  }
                  frame 12 {
                    # "This is the Initialize case"
                    n287 = call "Initialize and Enable.vi"("axis names"=string[] ["Y", "YY", "X", "Z", "U"]) -> ("error out"=w567:errorcluster, "controller out"=→"CONTROLLER":refnum<k24>)  [unwired: 5 in]
                    n288 = local write "error out"(w567) -> ()
                    n289 = Concatenate Strings(w571, "\r", ">", "Aerotech Initialized ") -> (w570:string)
                  }
                  frame 13 {
                    # "binary flag for only\nz homing, or home\nall axes"
                    # "just get z to 0"
                    # "home all axes"
                    # "This case determines\nwhether to home all\nor just bring the z to 0"
                    n290 = local read "CONTROLLER"() -> (w577:refnum<k24>)
                    n291 = Index Array(array=w583, index=0) -> (element=w581:dbl)
                    n292 = Not Equal To 0?(x=w581) -> (x != 0?=w580:bool)
                    n293 = Select(t="Z to 0 ", s=w580, f="Homing ") -> (s? t:f=w575:string)
                    n294 = call "Home Subvi.vi"("Only Z?"=w580, "controller in"=w577) -> ("error out"=w576:errorcluster)  [unwired: 4 in, 1 out]
                    n295 = Concatenate Strings(w587, "\r", ">", w575) -> (w586:string)
                    n296 = local write "Command log"(w586) -> ()
                    n297 = Concatenate Strings(w586, "-> Complete" ("string")) -> (w584:string)
                    n298 = local write "error out"(w576) -> ()
                  }
                  frame 14 {
                    # "position vector (corrected)"
                    # "memory or command\ncase"
                    # "slow or normal speed"
                    # "Add in any offset stored"
                    # "if the parameter is 0 use standard speed, otherwise use slow speed"
                    # "absolute or relative"
                    # "vector move case"
                    n299 = local read "Rotate State"() -> (w596:bool)
                    n300 = Index Array(array=w599, index=0) -> (element=w600:dbl)
                    n301 = Not Equal To 0?(x=w600) -> (x != 0?=w601:bool)
                    n302 = case shown="True" w601 {
                      tunnel: w599 -> [w629 w635]
                      tunnel: [w628 w632] -> w598
                      frame False {
                        n303 = Array Subset(array=w629, index=1, length=4) -> (w628:dbl[])
                      }
                      frame True {
                        n304 = local read "Stored Vectors"() -> (w636:T1[][])
                        n305 = Index Array(array=w635, index=1) -> (element=w634:dbl)
                        n306 = Index Array(array=w636, index (col)=w634) -> (element=w632:T1[])  [unwired: 1 in]
                      }
                    }
                    n307 = local read "Offset State"() -> (w597:bool)
                    n308 = Array To Spreadsheet String(delimiter (Tab)=", ", array=w598, 3:"%.3f" ("format string")) -> (spreadsheet string=w611:string)
                    n309 = case shown="False" w597 {
                      tunnel: w598 -> [w624 w627]
                      tunnel: [w624 w625] -> w595
                      frame False {
                        # "do nothing"
                      }
                      frame True {
                        # "offset\nvector"
                        n310 = local read "Offset"() -> (w626:dbl[])
                        n311 = Add(x=w626, y=w627) -> (x+y=w625:T1[])
                      }
                    }
                    n312 = case shown="True" w596 {
                      tunnel: w595 -> [w620 w622]
                      tunnel: [w620 w621] -> w594
                      frame False {
                        # "do nothing"
                      }
                      frame True {
                        n313 = local read "Rotation Offset"() -> (w623:dbl)
                        n314 = call "Rotate Offset.vi"("Input Vector"=w622, "theta"=w623) -> ("Output Vector"=w621:dbl[])  [unwired: 9 out]
                      }
                    }
                    n315 = local read "CONTROLLER"() -> (w593:refnum<k24>)
                    n316 = Index Array(array=w599, index #1=5 ("index"), index #2=6 ("index")) -> (element #1=w590:dbl, element #2=w603:dbl)
                    n317 = Not Equal To 0?(x=w603) -> (x != 0?=w592:bool)
                    n318 = Select(t="relative" ("string"), s=w592, f="absolute" ("string")) -> (s? t:f=w607:string)
                    n319 = Concatenate Strings(w614, "\r", ">", "Moving to: ", "\r", w611, "in " ("string"), w607) -> (w605:string)
                    n320 = local read "Angular Speed (deg/s"() -> (w618:dbl)
                    n321 = local write "Command log"(w605) -> ()
                    n322 = call "Vector Mover.vi"("Absolute/Relative (F/T)"=w592, "Movement Vector"=w594, "Angular Speed"=w618, "Vector Speed"=w590, "controller in"=w593) -> ("error out"=w591:errorcluster)  [unwired: 1 in, 3 out]
                    n323 = local write "error out"(w591) -> ()
                  }
                  frame 15 {
                    # "Camera Control"
                    # "enable the joystick"
                    n324 = Index Array(array=w647, index #1=0 ("index")) -> (element #1=w645:dbl)  [unwired: 1 in, 1 out]
                    n325 = Not Equal To 0?(x=w645) -> (x != 0?=w643:bool)
                    n326 = local read "Information"() -> (w640:T2)
                    n327 = And(x=w643, y=w642) -> (x .and. y?=w644:bool)
                    n328 = flat-sequence {
                      tunnel: [w659] -> w642
                      tunnel: [w658] -> w641
                      tunnel: w641 -> [w661]
                      tunnel: [w660] -> w639
                      frame #0 {
                        w659 = TRUE ("Joystick state")
                        n329 = local read "CONTROLLER"() -> (w658:refnum<k24>)
                        n330 = local write "Joystick state"(w659) -> ()
                      }
                      frame #1 {
                        n331 = call "Joystick Control.vi"("controller in"=w661) -> ("error out"=w660:errorcluster)  [unwired: 9 in, 1 out]
                      }
                      frame #2 {
                        n332 = local write "Joystick state"(FALSE ("Joystick state")) -> ()
                      }
                    }
                    n333 = case shown="False" w644 {
                      tunnel: [w667 w674] -> w638
                      tunnel: w640 -> [w664 w680]
                      frame False {
                        n334 = while {
                          tunnel: [w669] -> w666
                          tunnel: w664 -> [w668]
                          tunnel: [w668] -> w663
                          stop <- w672 stop-if-true
                          n335 = local read "Joystick state"() -> (w671:bool)
                          n336 = Not(x=w671) -> (.not. x?=w670:bool)
                          n337 = call "Vision Acquisition2"("Stop (F)"=w670) -> ("Image Out"=w669:T4, "Stopped"=w672:bool)  [unwired: 24 in, 1 out]
                          "Image Out" <- w669
                        }
                        n338 = local write "Information"(T2."Camera Image 2" ("Information")) -> ()
                        n339 = call "IMAQ Dispose"("Image"=w666) -> ()  [unwired: 5 in, 1 out]
                        n340 = local read "error out"() -> (w667:errorcluster)
                        n341 = local write "Information"(w663) -> ()
                      }
                      frame True {
                        n342 = while {
                          tunnel: w680 -> [w692]
                          tunnel: [w692] -> w679
                          tunnel: [FALSE] -> w678
                          tunnel: [w683] -> w675
                          tunnel: [w682] -> w676
                          stop <- w689 stop-if-true
                          # "flips and add crosshair"
                          n343 = local read "Joystick state"() -> (w690:bool)
                          n344 = event shown="[1] \"Zoomtofit\": Value Change" {
                            selector: _ -> [_ _]
                            dyn-events: _ -> [_ _]
                            timeout: 50 -> [_ _]
                            tunnel: [FALSE ("Zoomtofit") TRUE ("Zoomtofit")] -> w687
                            event Timeout {
                              n345 = event-data() -> ()  [unwired: 3 out]
                            }
                            event "Zoomtofit": Value Change {
                              n346 = event-data() -> ()  [unwired: 3 out]
                              n347 = local write "Zoomtofit"(FALSE ("Zoomtofit")) -> ()
                            }
                          }
                          n348 = Not(x=w690) -> (.not. x?=w688:bool)
                          n349 = call "Vision Acquisition"("Stop (F)"=w688) -> ("Image Out"=w685:T4, "Stopped"=w689:bool, "error out"=w684:errorcluster)  [unwired: 24 in]
                          n350 = property on="Image" class="ImageControl"("Zoom to Fit Mode"=w687) -> ()  [unwired: 2 in, 2 out]
                          n351 = call "Image Process mk2.vi"("error in"=w684, "Image"=w685) -> ("error out"=w683:errorcluster, "Image Out"=w682:T4)  [unwired: 2 in]
                          "Image" <- w682
                          n352 = Wait Until Next ms Multiple(millisecond multiple=u32 200) -> ()  [unwired: 1 out]
                        }
                        n353 = local write "Information"(T5."Camera Image" ("Information")) -> ()
                        n354 = call "IMAQ Dispose"("Image"=w676, "error in (no error)"=w675) -> ("error out"=w674:errorcluster)  [unwired: 4 in]
                        n355 = local write "Information"(w679) -> ()
                        n356 = property on="Zoomtofit" class="Bool (strict)"("Visible"=w678) -> ()  [unwired: 2 in, 2 out]
                        n357 = property on="Zoomtofit" class="Bool (strict)"("Visible"=FALSE) -> ()  [unwired: 2 in, 2 out]
                      }
                    }
                    n358 = Concatenate Strings(w654, "\r", ">", "JoyStick Control Active ", "\r", "Buttons; A->Vert/Horiz, B ->Slow/Fast, C->End/Ack" ("string")) -> (w651:string)
                    n359 = local write "Command log"(w651) -> ()
                    n360 = Merge Errors(w638, w639) -> (w637:errorcluster)
                    n361 = local write "error out"(w637) -> ()
                    n362 = Concatenate Strings(w651, "\r", "Joystick Released" ("string")) -> (w648:string)
                  }
                  frame 16 {
                    # "Store Offset for use in vector move commands"
                    # "Set offset Vector"
                    n363 = local write "Offset"(w696) -> ()
                    n364 = Array To Spreadsheet String(delimiter (Tab)=",", array=w696, 3:"%f" ("format string")) -> (spreadsheet string=w697:string)
                    n365 = Concatenate Strings(w702, "\r", ">", "Offset set to: ", "\r", w697) -> (w701:string)
                  }
                  frame 17 {
                    # "When the got to command is issued, the previous command line \nwill be changed to white to update the high lighted position within \nthe command table."
                    # "Lets user move to any command number in the command array"
                    # "Goto command"
                    n366 = Index Array(array=w710, index=0) -> (element=w706:dbl)
                    n367 = Number To Decimal String(number=w706, width (-)=i16 2) -> (decimal integer string=w707:string)
                    n368 = flat-sequence {
                      tunnel: w706 -> [w722]
                      frame #0 {
                        n369 = local read "Current Command number"() -> (w718:dbl)
                        n370 = control-ref of="Command Table"() -> (w719:refnum<vi>)
                        n371 = Add(x=1.0, y=w718) -> (x+y=w717:dbl)
                        n372 = call "Color row of table.vi"("Edit Line"=w717, "Number of Columns"=11, "Color"=u32 16448250, "Table in"=w719) -> ()  [unwired: 7 in, 1 out]
                      }
                      frame #1 {
                        n373 = local write "Current Command number"(w722) -> ()
                      }
                    }
                    n374 = Concatenate Strings(w712, "\r", ">", "Going to line:  ", w707) -> (w711:string)
                  }
                  frame 18 {
                    # "convert to bool"
                    # "Control Vacuums"
                    n375 = for {
                      N: 3 -> [_]
                      tunnel: w732 -> [w741] mode=indexing
                      tunnel: [w740] -> w731 mode=indexing
                      tunnel: [w737] -> w728 mode=indexing
                      n376 = Not Equal To 0?(x=w741) -> (x != 0?=w740:bool)
                      n377 = Select(t=1.0, s=w740, f=0.0) -> (s? t:f=w737:dbl)
                    }
                    n378 = Array To Spreadsheet String(delimiter (Tab)=", ", array=w728, 3:"%d" ("format string")) -> (spreadsheet string=w724:string)
                    n379 = call "Pressure Controller Gantry Head.vi"("Pressure Controls"=w731) -> ("Output status of pressure lines"=w729:bool[])  [unwired: 1 in, 9 out]
                    n380 = local write "Gantry Head"(w729) -> ()
                    n381 = Concatenate Strings(w734, "\r", ">", "Pressures On Gantry Head Set to:  ", "\r", w724) -> (w733:string)
                  }
                  frame 19 {
                    # "Enable or disable needle pressure"
                    n382 = Index Array(array=w748, index=0) -> (element=w746:dbl)
                    n383 = Not Equal To 0?(x=w746) -> (x != 0?=w742:bool)
                    n384 = call "Needle Pressure Control.vi"("Needle State"=w742) -> ()  [unwired: 1 in, 10 out]
                    n385 = Select(t="enabled.", s=w742, f="disabled.") -> (s? t:f=w743:string)
                    n386 = Concatenate Strings(w750, "\r", ">", "Needle pressure ", w743) -> (w749:string)
                    n387 = local write "Needle Pressure State"(w742) -> ()
                  }
                  frame 20 {
                    # "flipped large case structure and smaller case structure"
                    # "Store a point, either from current position or from command menu"
                    n388 = local read "Stored Vectors"() -> (w764:T1[][])
                    n389 = Index Array(array=w755, index #1=0 ("index"), index #2=1 ("index")) -> (element #1=w754:dbl, element #2=w766:dbl)
                    n390 = Not Equal To 0?(x=w766) -> (x != 0?=w765:bool)
                    n391 = Number To Decimal String(number=w754, width (-)=i16 3) -> (decimal integer string=w758:string)
                    n392 = case shown="False" w765 {
                      tunnel: [w776 w790] -> w760
                      tunnel: w755 -> [w781 w793]
                      frame False {
                        # "take parameters\nand store"
                        n393 = Array Subset(array=w781, index=2, length=5) -> (w775:dbl[])
                        n394 = Index Array(array=w775, index=4) -> (element=w778:dbl)
                        n395 = Not Equal To 0?(x=w778) -> (x != 0?=w777:bool)
                        n396 = case shown="True" w777 {
                          tunnel: [w784 w786] -> w776
                          tunnel: w775 -> [w785 w789]
                          frame False {
                            n397 = Array Subset(array=w785, index=0, length=4) -> (w784:dbl[])
                          }
                          frame True {
                            n398 = Array Subset(array=w789, index=0, length=2) -> (w786:dbl[])
                          }
                        }
                      }
                      frame True {
                        # "take current position"
                        n399 = Index Array(array=w793, index=6) -> (element=w792:dbl)
                        n400 = Not Equal To 0?(x=w792) -> (x != 0?=w791:bool)
                        n401 = case shown="True" w791 {
                          tunnel: [w795 w796] -> w790
                          frame False {
                            n402 = local read "Current Position"() -> (w795:dbl[])
                          }
                          frame True {
                            n403 = local read "Current Position"() -> (w797:dbl[])
                            n404 = Array Subset(array=w797, index=0, length=2) -> (w796:dbl[])
                          }
                        }
                      }
                    }
                    n405 = Array To Spreadsheet String(delimiter (Tab)=",", array=w760, 3:"%.3f" ("format string")) -> (spreadsheet string=w756:string)
                    n406 = Concatenate Strings(w770, "\r", ">", "Point Stored to slot: ", w758, "\r", w756) -> (w769:string)
                    n407 = Replace Array Subset(array=w764, new element=w760, index (col)=w754) -> (w763:T1[][])  [unwired: 1 in]
                    n408 = local write "Stored Vectors"(w763) -> ()
                  }
                  frame 21 {
                    # "Set offset state"
                    n409 = Index Array(array=w803, index=0) -> (element=w801:dbl)
                    n410 = Not Equal To 0?(x=w801) -> (x != 0?=w800:bool)
                    n411 = local write "Offset State"(w800) -> ()
                    n412 = Select(t="enabled.", s=w800, f="disabled.") -> (s? t:f=w811:string)
                    n413 = Concatenate Strings(w805, "\r", ">", "Offset ", w811) -> (w804:string)
                  }
                  frame 22 {
                    # "only lateral"
                    # "store to vectors"
                    # "Calculate center"
                    # "Find Center from 2 points"
                    n414 = local read "Stored Vectors"() -> (w830:T1[][])
                    n415 = Index Array(array=w831) -> (element #1=w823:dbl, element #2=w822:dbl, element #3=w824:dbl)  [unwired: 3 in]
                    n416 = Index Array(array=w830, index (col) #1=w823, index (col) #2=w822) -> (element #1=w821:T1[], element #2=w820:T1[])  [unwired: 2 in]
                    n417 = Add(x=w821, y=w820) -> (x+y=w818:T1[])
                    n418 = Divide(x=w818, y=2.0) -> (x/y=w817:T1[])
                    n419 = Array Subset(array=w817, index=0, length=2) -> (w812:T1[])
                    n420 = Number To Decimal String(number=w824, width (-)=i16 1) -> (decimal integer string=w825:string)
                    n421 = Concatenate Strings(w835, "\r", ">", "Center stored to slot: ", w825) -> (w834:string)
                    n422 = local read "Stored Vectors"() -> (w829:T1[][])
                    n423 = Build Array (concatenate)(w812, 0.0 ("element"), 0.0 ("element")) -> (w828:T1[])
                    n424 = Replace Array Subset(array=w829, new element=w828, index (col)=w824) -> (w827:T1[][])  [unwired: 1 in]
                    n425 = local write "Stored Vectors"(w827) -> ()
                  }
                  frame 23 {
                    # "only lateral"
                    # "final - initial"
                    # "first start then finish"
                    # "find distance between two points and store it"
                    n426 = local read "Stored Vectors"() -> (w851:T1[][])
                    n427 = Index Array(array=w852) -> (element #1=w850:dbl, element #2=w849:dbl, element #3=w842:dbl)  [unwired: 3 in]
                    n428 = Index Array(array=w851, index (col) #1=w850, index (col) #2=w849) -> (element #1=w847:T1[], element #2=w848:T1[])  [unwired: 2 in]
                    n429 = Subtract(x=w848, y=w847) -> (x-y=w846:T1[])
                    n430 = Array Subset(array=w846, index=0, length=2) -> (w839:T1[])
                    n431 = local read "Stored Vectors"() -> (w843:T1[][])
                    n432 = Build Array (concatenate)(w839, 0.0 ("element"), 0.0 ("element")) -> (w838:T1[])
                    n433 = Number To Decimal String(number=w842, width (-)=i16 1) -> (decimal integer string=w859:string)
                    n434 = Concatenate Strings(w855, "\r", ">", "Distance stored to slot: ", w859) -> (w854:string)
                    n435 = Replace Array Subset(array=w843, new element=w838, index (col)=w842) -> (w837:T1[][])  [unwired: 1 in]
                    n436 = local write "Stored Vectors"(w837) -> ()
                  }
                  frame 24 {
                    w865 = 0.0 ("element")
                    w868 = 2 ("length")
                    w869 = 0 ("index")
                    # "in Degrees"
                    # "store new vector"
                    # "make vector with offset"
                    # "retrieve storage vectors"
                    # "from storage"
                    # "lateral only"
                    # "calculate angular offset between two vectors"
                    n437 = Index Array(array=w884, index #1=0 ("index"), index #2=1 ("index")) -> (element #1=w880:dbl, element #2=w879:dbl, element #3=w860:dbl)  [unwired: 1 in]
                    n438 = local read "Stored Vectors"() -> (w881:T1[][])
                    n439 = Index Array(array=w881, index (col) #1=w880, index (col) #2=w879) -> (element #1=w871:T1[], element #2=w870:T1[])  [unwired: 2 in]
                    n440 = Array Subset(array=w871, index=w869, length=w868) -> (w867:T1[])
                    n441 = Array Subset(array=w870, index=w869, length=w868) -> (w866:T1[])
                    n442 = call "2d angular offset.vi"("Vector 2"=w866, "Vector 1"=w867) -> ("Offset Angle"=w864:dbl)  [unwired: 9 out]
                    n443 = Build Array(w865, w865, w865, w864) -> (w863:dbl[])
                    n444 = local read "Stored Vectors"() -> (w862:T1[][])
                    n445 = Replace Array Subset(array=w862, new element=w863, index (col)=w860) -> (w861:T1[][])  [unwired: 1 in]
                    n446 = Number To Decimal String(number=w860, width (-)=i16 1) -> (decimal integer string=w874:string)
                    n447 = Concatenate Strings(w873, "\r", ">", "Angle offset stored to slot: ", w874) -> (w872:string)
                    n448 = local write "Stored Vectors"(w861) -> ()
                  }
                  frame 25 {
                    # "This block stops it once the touch switch is active"
                    # "move down a max of 8mm"
                    # "move to touch on the z axis"
                    n449 = local read "CONTROLLER"() -> (w886:refnum<k24>)
                    n450 = call "Vector Mover.vi"("Absolute/Relative (F/T)"=TRUE, "Movement Vector"=dbl[] [0.0, 0.0, 8.0, 0.0, 0.0], "Angular Speed"=1.0, "Vector Speed"=0.05, "controller in"=w886) -> ("error out"=w885:errorcluster)  [unwired: 1 in, 3 out]
                    n451 = flat-sequence {
                      frame #0 {
                        n452 = while {
                          stop <- w896 stop-if-true
                          n453 = call "Touch and Limit controller.vi"() -> ("Touching"=w896:bool)  [unwired: 1 in, 4 out]
                          n454 = Wait (ms)(milliseconds to wait=u32 50) -> ()  [unwired: 1 out]
                        }
                      }
                      frame #1 {
                        n455 = local read "CONTROLLER"() -> (w898:refnum<k24>)
                        n456 = call "Abort All Movement.vi"("controller in"=w898) -> ()  [unwired: 9 in, 2 out]
                      }
                    }
                    n457 = local write "error out"(w885) -> ()
                    n458 = Concatenate Strings(w892, "\r", ">", "Moving until touch Z. ") -> (w891:string)
                  }
                  frame 26 {
                    # "still need a commmand to set rotation angle, but planned for later"
                    # "enable rotation offset"
                    n459 = Index Array(array=w904, index=0) -> (element=w902:dbl)
                    n460 = Not Equal To 0?(x=w902) -> (x != 0?=w899:bool)
                    n461 = local write "Rotate State"(w899) -> ()
                    n462 = Select(t="enabled.", s=w899, f="disabled.") -> (s? t:f=w901:string)
                    n463 = Concatenate Strings(w906, "\r", ">", "Rotation offset ", w901) -> (w905:string)
                  }
                  frame 27 {
                    # "grab the angle\nonly from vector"
                    # "store rotation from stored vectors"
                    n464 = Index Array(array=w918, index=0) -> (element=w911:dbl)
                    n465 = local read "Stored Vectors"() -> (w916:T1[][])
                    n466 = Index Array(array=w916, index (row)=3 ("disabled index (row)"), index (col)=w911) -> (element=w914:T1)
                    n467 = local write "Rotation Offset"(w914) -> ()
                    n468 = Number To Decimal String(number=w911, width (-)=i16 1) -> (decimal integer string=w913:string)
                    n469 = Concatenate Strings(w920, "\r", ">", "Angle taken from slot ", w913) -> (w919:string)
                  }
                  frame 28 {
                    w936 = 0.0 ("element")
                    # "Change the coordinates CAMERA no longer flips the image"
                    # "template file"
                    # "store new vector"
                    # "Pattern Recognition Case"
                    n470 = Index Array(array=w929, index=2) -> (element=w928:dbl)
                    n471 = Index Array(array=w929, index=1) -> (element=w938:dbl)
                    n472 = call "Pat Match Full.vi"("Minimum Match Score"=w928, "Template File Path"=path "C:/Users/Admin/Desktop/Main_Module_Assembly/Pattern recognition/templates/color.png") -> ("Matched?"=w934:bool, "Score"=→"Match Score":dbl, "x rel move"=w924:dbl, "y rel move"=w925:dbl)  [unwired: 9 in, 1 out]
                    n473 = Select(t="Found", s=w934, f="Failed") -> (s? t:f=w933:string)
                    n474 = Concatenate Strings(w942, "\r", ">", "Pattern Matching: ", w933) -> (w935:string)
                    n475 = Build Array(w925, w924, w936, w936) -> (w941:dbl[])
                    n476 = local read "Stored Vectors"() -> (w940:T1[][])
                    n477 = Replace Array Subset(array=w940, new element=w941, index (col)=w938) -> (w937:T1[][])  [unwired: 1 in]
                    n478 = local write "Stored Vectors"(w937) -> ()
                  }
                  frame 29 {
                    # "convert to numbers"
                    # "get index row"
                    # "Vector move to Index point"
                    n479 = local read "Index Points"() -> (w963:string[][])
                    n480 = Index Array(array=w965, index #1=0 ("index"), index #2=1 ("index")) -> (element #1=w962:dbl, element #2=w956:dbl)
                    n481 = Index Array(array=w963, index (row)=w962) -> (element=w961:string[])  [unwired: 1 in]
                    n482 = Split 1D Array(array=w961, index=3) -> (first subarray=w948:string[], second subarray=w959:string[])
                    n483 = Index Array(array=w948, index=1) -> (element=w947:string)
                    n484 = for {
                      tunnel: w959 -> [w968] mode=indexing
                      tunnel: [w967] -> w958 mode=indexing
                      n485 = Fract/Exp String To Number(string=w968) -> (number=w967:dbl)  [unwired: 3 in, 1 out]
                    }
                    n486 = local read "CONTROLLER"() -> (w966:refnum<k24>)
                    n487 = call "Vector Mover.vi"("Absolute/Relative (F/T)"=FALSE, "Movement Vector"=w958, "Angular Speed"=2.0, "Vector Speed"=w956, "controller in"=w966) -> ()  [unwired: 1 in, 4 out]
                    n488 = Concatenate Strings(w950, "\r", ">", "Moving to Index point:  ", w947) -> (w946:string)
                    n489 = local write "Command log"(w946) -> ()
                  }
                  frame 30 {
                    # "Vacuum control"
                    # "convert to bool"
                    n490 = for {
                      N: 4 -> [_]
                      tunnel: w971 -> [w987] mode=indexing
                      tunnel: [w986] -> w980 mode=indexing
                      tunnel: [w983] -> w978 mode=indexing
                      n491 = Not Equal To 0?(x=w987) -> (x != 0?=w986:bool)
                      n492 = Select(t=1.0, s=w986, f=0.0) -> (s? t:f=w983:dbl)
                    }
                    n493 = Array To Spreadsheet String(delimiter (Tab)=", ", array=w978, 3:"%d" ("format string")) -> (spreadsheet string=w974:string)
                    n494 = Concatenate Strings(w972, "\r", ">", "Pressures on Station C Set to:  ", "\r", w974) -> (w970:string)
                    n495 = call "Pressure Control Base Plate 2.vi"("Pressure Controls"=w980) -> ("Output status of pressure lines"=→"Station C":bool[])  [unwired: 9 in, 1 out]
                  }
                  frame 31 {
                    # "Controls Vacuum for the right base plate, currently denoted Base Plate 1."
                    # "convert to bool"
                    n496 = for {
                      N: 4 -> [_]
                      tunnel: w992 -> [w1006] mode=indexing
                      tunnel: [w1005] -> w989 mode=indexing
                      tunnel: [w1002] -> w998 mode=indexing
                      n497 = Not Equal To 0?(x=w1006) -> (x != 0?=w1005:bool)
                      n498 = Select(t=1.0, s=w1005, f=0.0) -> (s? t:f=w1002:dbl)
                    }
                    n499 = Array To Spreadsheet String(delimiter (Tab)=", ", array=w998, 3:"%d" ("format string")) -> (spreadsheet string=w994:string)
                    n500 = call "Pressure Control Base Plate 1.vi"("Pressure Controls"=w989) -> ("Output status of pressure lines"=→"Station D":bool[])  [unwired: 9 in, 1 out]
                    n501 = Concatenate Strings(w991, "\r", ">", "Pressures on Station D Set to:  ", "\r", w994) -> (w990:string)
                  }
                  frame 32 {
                    # "Controls the EFD Ultimus by turning on the pressure. Purposed for Encapsulation."
                    n502 = Index Array(array=w1011, index=0) -> (element=w1010:dbl)
                    n503 = Not Equal To 0?(x=w1010) -> (x != 0?=w1009:bool)
                    n504 = call "Encapsulation_Control.vi"("Encapsulation  State"=w1009) -> ()  [unwired: 10 in, 1 out]
                    n505 = Select(t="enabled.", s=w1009, f="disabled.") -> (s? t:f=w1018:string)
                    n506 = Concatenate Strings(w1007, "\r", ">", "Encapsulation:  ", w1018) -> (w1008:string)
                    n507 = local write "Encapsulation Pressure"(w1009) -> ()
                  }
                  frame 33 {
                    # "Calculates a 3D difference vector, as opposed to command 23 which only calculates the distance in X and Y."
                    # "final - initial"
                    n508 = local read "Stored Vectors"() -> (w1033:T1[][])
                    n509 = Index Array(array=w1040) -> (element #1=w1035:dbl, element #2=w1034:dbl, element #3=w1019:dbl)  [unwired: 3 in]
                    n510 = Index Array(array=w1033, index (col) #1=w1035, index (col) #2=w1034) -> (element #1=w1038:T1[], element #2=w1039:T1[])  [unwired: 2 in]
                    n511 = Subtract(x=w1039, y=w1038) -> (x-y=w1037:T1[])
                    n512 = Array Subset(array=w1037, index=0, length=3) -> (w1030:T1[])
                    n513 = local read "Stored Vectors"() -> (w1031:T1[][])
                    n514 = Build Array (concatenate)(w1030, 0.0) -> (w1029:T1[])
                    n515 = Replace Array Subset(array=w1031, new element=w1029, index (col)=w1019) -> (w1027:T1[][])  [unwired: 1 in]
                    n516 = Number To Decimal String(number=w1019, width (-)=i16 1) -> (decimal integer string=w1026:string)
                    n517 = Concatenate Strings(w1022, "\r", ">", "3D Vector stored to slot: ", w1026) -> (w1021:string)
                    n518 = local write "Stored Vectors"(w1027) -> ()
                  }
                  frame 34 {
                    # "Sets the offset vector from a point in the stored vectors array."
                    n519 = Index Array(array=w1043, index=0) -> (element=w1042:dbl)
                    n520 = local read "Stored Vectors"() -> (w1045:T1[][])
                    n521 = Index Array(array=w1045, index (col)=w1042) -> (element=w1041:T1[])  [unwired: 1 in]
                    n522 = local write "Offset"(w1041) -> ()
                    n523 = Array To Spreadsheet String(delimiter (Tab)=",", array=w1041, 3:"%f" ("format string")) -> (spreadsheet string=w1048:string)
                    n524 = Concatenate Strings(w1047, "\r", ">", "Offset set to: ", "\r", w1048) -> (w1046:string)
                  }
                  frame 35 {
                    # "Adds a vector to an existing vector in the Stored Vectors Array."
                    n525 = Index Array(array=w1069) -> (element #1=w1068:dbl, element #2=w1067:dbl, element #3=w1066:dbl, element #4=w1061:dbl, element #5=w1060:dbl, element #6=w1065:dbl)  [unwired: 6 in]
                    n526 = Build Array(w1068, w1067, w1066, w1061) -> (w1058:dbl[])
                    n527 = local read "Stored Vectors"() -> (w1074:T1[][])
                    n528 = Index Array(array=w1074, index (col)=w1060) -> (element=w1073:T1[])  [unwired: 1 in]
                    n529 = Add(x=w1058, y=w1073) -> (x+y=w1071:T1[])
                    n530 = Array To Spreadsheet String(delimiter (Tab)=",", array=w1058, 3:"%6f" ("format string")) -> (spreadsheet string=w1063:string)
                    n531 = local read "Stored Vectors"() -> (w1072:T1[][])
                    n532 = Number To Decimal String(number=w1065) -> (decimal integer string=w1055:string)  [unwired: 1 in]
                    n533 = Number To Decimal String(number=w1060) -> (decimal integer string=w1059:string)  [unwired: 1 in]
                    n534 = Replace Array Subset(array=w1072, new element=w1071, index (col)=w1065) -> (w1070:T1[][])  [unwired: 1 in]
                    n535 = local write "Stored Vectors"(w1070) -> ()
                    n536 = Concatenate Strings(w1076, "\r", ">", "Vector: ", w1063, "  ,added to slot: " ("string"), w1059, "            Stored in slot: " ("string"), w1055) -> (w1075:string)
                  }
                  frame 36 {
                    # "Scales a Vector by a number"
                    n537 = local read "Stored Vectors"() -> (w1092:T1[][])
                    n538 = Index Array(array=w1095, index #1=0 ("index"), index #2=1 ("index"), index #3=2 ("index")) -> (element #1=w1084:dbl, element #2=w1091:dbl, element #3=w1085:dbl)
                    n539 = Index Array(array=w1092, index (col)=w1091) -> (element=w1090:T1[])  [unwired: 1 in]
                    n540 = Multiply(x=w1084, y=w1090) -> (x*y=w1086:T1[])
                    n541 = local read "Stored Vectors"() -> (w1088:T1[][])
                    n542 = Number To Decimal String(number=w1085) -> (decimal integer string=w1082:string)  [unwired: 1 in]
                    n543 = Replace Array Subset(array=w1088, new element=w1086, index (col)=w1085) -> (w1087:T1[][])  [unwired: 1 in]
                    n544 = Number To Decimal String(number=w1084) -> (decimal integer string=w1080:string)  [unwired: 1 in]
                    n545 = Concatenate Strings(w1099, "\r", ">" ("string"), "Vector in slot:  " ("string"), w1082, "      Scaled By: " ("string"), w1080) -> (w1096:string)
                    n546 = local write "Stored Vectors"(w1087) -> ()
                  }
                  frame 37 {
                    # "3D Midpoint of Vector"
                    # "Calculate center"
                    n547 = local read "Stored Vectors"() -> (w1107:T1[][])
                    n548 = Index Array(array=w1108) -> (element #1=w1123:dbl, element #2=w1122:dbl, element #3=w1101:dbl)  [unwired: 3 in]
                    n549 = Index Array(array=w1107, index (col) #1=w1123, index (col) #2=w1122) -> (element #1=w1121:T1[], element #2=w1120:T1[])  [unwired: 2 in]
                    n550 = Add(x=w1121, y=w1120) -> (x+y=w1118:T1[])
                    n551 = Divide(x=w1118, y=2.0) -> (x/y=w1117:T1[])
                    n552 = Array Subset(array=w1117, index=0, length=3) -> (w1103:T1[])
                    n553 = local read "Stored Vectors"() -> (w1104:T1[][])
                    n554 = Build Array (concatenate)(w1103, 0.0 ("element")) -> (w1102:T1[])
                    n555 = Number To Decimal String(number=w1101, width (-)=i16 1) -> (decimal integer string=w1110:string)
                    n556 = Concatenate Strings(w1109, "\r", ">", "3D Center stored to slot: ", w1110) -> (w1100:string)
                    n557 = Replace Array Subset(array=w1104, new element=w1102, index (col)=w1101) -> (w1105:T1[][])  [unwired: 1 in]
                    n558 = local write "Stored Vectors"(w1105) -> ()
                  }
                  frame 38 {
                    # "Re-Intializes the Stored Vector Array"
                    n559 = Initialize Array(0.0 ("element"), 4 ("dimension size"), 500 ("dimension size")) -> (w1129:dbl[][])
                    n560 = local write "Stored Vectors"(w1129) -> ()
                    n561 = Concatenate Strings(w1125, "\r", ">", "Stored Vectors Array Cleared ") -> (w1124:string)
                  }
                  frame 39 {
                    # "convert to bool"
                    n562 = for {
                      N: 4 -> [_]
                      tunnel: [w1151] -> w1137 mode=indexing
                      tunnel: [w1148] -> w1143 mode=indexing
                      tunnel: w1135 -> [w1147] mode=indexing
                      n563 = Not Equal To 0?(x=w1147) -> (x != 0?=w1151:bool)
                      n564 = Select(t=1.0, s=w1151, f=0.0) -> (s? t:f=w1148:dbl)
                    }
                    n565 = Array To Spreadsheet String(delimiter (Tab)=", ", array=w1143, 3:"%d" ("format string")) -> (spreadsheet string=w1139:string)
                    n566 = call "Pressure Control Base Plate 1 Double 2.vi"("Pressure Controls"=w1137) -> ("Output status of pressure lines"=→"Station B":bool[])  [unwired: 9 in, 1 out]
                    n567 = Concatenate Strings(w1136, "\r", ">", "Pressures on Station B Set to:  ", "\r", w1139) -> (w1133:string)
                  }
                  frame 40 {
                    # "convert to bool"
                    n568 = for {
                      N: 4 -> [_]
                      tunnel: [w1170] -> w1156 mode=indexing
                      tunnel: [w1167] -> w1162 mode=indexing
                      tunnel: w1154 -> [w1166] mode=indexing
                      n569 = Not Equal To 0?(x=w1166) -> (x != 0?=w1170:bool)
                      n570 = Select(t=1.0, s=w1170, f=0.0) -> (s? t:f=w1167:dbl)
                    }
                    n571 = Array To Spreadsheet String(delimiter (Tab)=", ", array=w1162, 3:"%d" ("format string")) -> (spreadsheet string=w1158:string)
                    n572 = call "Pressure Control Base Plate 2 Double 2.vi"("Pressure Controls"=w1156) -> ("Output status of pressure lines"=→"Station A":bool[])  [unwired: 9 in, 1 out]
                    n573 = Concatenate Strings(w1155, "\r", ">", "Pressures on Station A Set to:  ", "\r", w1158) -> (w1152:string)
                  }
                  frame 41 {
                    # "convert to bool"
                    n574 = for {
                      N: 4 -> [_]
                      tunnel: [w1189] -> w1173 mode=indexing
                      tunnel: [w1186] -> w1181 mode=indexing
                      tunnel: w1174 -> [w1185] mode=indexing
                      n575 = Not Equal To 0?(x=w1185) -> (x != 0?=w1189:bool)
                      n576 = Select(t=1.0, s=w1189, f=0.0) -> (s? t:f=w1186:dbl)
                    }
                    n577 = Array To Spreadsheet String(delimiter (Tab)=", ", array=w1181, 3:"%d" ("format string")) -> (spreadsheet string=w1177:string)
                    n578 = call "Pressure Control StationE.vi"("Pressure Controls"=w1173) -> ("Output status of pressure lines"=→"Station E":bool[])  [unwired: 9 in, 1 out]
                    n579 = Concatenate Strings(w1175, "\r", ">", "Pressures on Station E Set to:  ", "\r", w1177) -> (w1172:string)
                  }
                  frame 42 {
                    # "convert to bool"
                    n580 = for {
                      N: 4 -> [_]
                      tunnel: [w1208] -> w1191 mode=indexing
                      tunnel: [w1205] -> w1200 mode=indexing
                      tunnel: w1192 -> [w1204] mode=indexing
                      n581 = Not Equal To 0?(x=w1204) -> (x != 0?=w1208:bool)
                      n582 = Select(t=1.0, s=w1208, f=0.0) -> (s? t:f=w1205:dbl)
                    }
                    n583 = Array To Spreadsheet String(delimiter (Tab)=", ", array=w1200, 3:"%d" ("format string")) -> (spreadsheet string=w1196:string)
                    n584 = call "Pressure Control StationF.vi"("Pressure Controls"=w1191) -> ("Output status of pressure lines"=→"Station F":bool[])  [unwired: 9 in, 1 out]
                    n585 = Concatenate Strings(w1194, "\r", ">", "Pressures on Station F Set to:  ", "\r", w1196) -> (w1193:string)
                  }
                  frame 43 {
                    # "Autofocus Case"
                    n586 = local read "CONTROLLER"() -> (w1210:refnum<k24>)
                    n587 = call "Autofocus.vi"("controller in"=w1210) -> ("Image Out 2"=w1209:T4)  [unwired: 9 in, 1 out]
                    n588 = local write "Image"(w1209) -> ()
                    n589 = Concatenate Strings(w1212, "\r", ">", "Auto focus complete  ") -> (w1211:string)
                  }
                  frame 44 {
                    n590 = Index Array(array=w1216, index=0) -> (element=w1217:dbl)
                    n591 = case shown="2" w1217 {
                      tunnel: w1220 -> [w1221 w1228 w1241 w1252 w1262 w1279 w1293 w1306]
                      tunnel: [w1221 w1227 w1240 w1251 w1261 w1278 w1292 w1305] -> w1219
                      tunnel: w1216 -> [_ w1226 _ _ _ w1274 _ w1304]
                      frame 0, Default {
                      }
                      frame 1 {
                        # "template file"
                        # "Sensor Pattern Recognition Case"
                        n592 = local read "CONTROLLER"() -> (w1222:refnum<k24>)
                        n593 = Index Array(array=w1226, index=2) -> (element=w1225:dbl)
                        n594 = call "Pat Match Full with Move.vi"("Minimum Match Score"=w1225, "Template File Path"=path "C:/Users/Admin/Desktop/Main_Module_Assembly/Pattern recognition/templates/color.png", "controller in"=w1222) -> ("Matched?"=w1224:bool, "Score"=w1223:dbl)  [unwired: 8 in, 3 out]
                        "Matched?" <- w1224
                        n595 = Select(t="Found", s=w1224, f="Failed") -> (s? t:f=w1233:string)
                        n596 = Concatenate Strings(w1228, "\r", ">", "Pattern Matching with Move: ", w1233) -> (w1227:string)
                        n597 = local write "Match Score"(w1223) -> ()
                      }
                      frame 2 {
                        # "Creates vector vector for relative movements"
                        # "HDI TR Pattern Recognition Case"
                        n598 = local read "CONTROLLER"() -> (w1239:refnum<k24>)
                        n599 = call "HDI Pat Match Full with Move TR.vi"("controller in"=w1239) -> ("In Range?"=w1238:bool, "Horizontal vector"=→"Vertical vector":dbl[])  [unwired: 10 in, 3 out]
                        "In Range?" <- w1238
                        n600 = Select(t="Found", s=w1238, f="Failed") -> (s? t:f=w1244:string)
                        n601 = Concatenate Strings(w1241, "\r", ">", "Pattern Matching with Move: ", w1244) -> (w1240:string)
                      }
                      frame 3 {
                        # "HDI TL Pattern Recognition Case"
                        n602 = local read "CONTROLLER"() -> (w1250:refnum<k24>)
                        n603 = call "HDI Pat Match Full with Move TL.vi"("controller in"=w1250) -> ("In Range?"=w1249:bool, "Vertical vector"=w1248:dbl[])  [unwired: 10 in, 3 out]
                        n604 = Select(t="Found", s=w1249, f="Failed") -> (s? t:f=w1255:string)
                        n605 = Concatenate Strings(w1252, "\r", ">", "Pattern Matching with Move: ", w1255) -> (w1251:string)
                        n606 = local write "Vertical vector"(w1248) -> ()
                        n607 = local write "In Range?"(w1249) -> ()
                      }
                      frame 4 {
                        # "HDI BL Pattern Recognition Case"
                        n608 = local read "CONTROLLER"() -> (w1260:refnum<k24>)
                        n609 = call "HDI Pat Match Full with Move BL.vi"("controller in"=w1260) -> ("In Range?"=w1259:bool)  [unwired: 11 in, 3 out]
                        n610 = Select(t="Found", s=w1259, f="Failed") -> (s? t:f=w1265:string)
                        n611 = Concatenate Strings(w1262, "\r", ">", "Pattern Matching with Move: ", w1265) -> (w1261:string)
                        n612 = local write "In Range?"(w1259) -> ()
                      }
                      frame 5 {
                        # "HDI BL Pattern Recognition Case"
                        n613 = Index Array(array=w1274, index #1=3 ("index"), index #2=4 ("index")) -> (element #1=w1272:dbl, element #2=w1269:dbl)
                        n614 = case shown="1" w1272 {
                          tunnel: [w1288 w1289] -> w1271
                          frame 0, Default {
                            w1288 = u32 1 items=["Left to Right", "Right to Left", "Top to Bottom", "Bottom to Top"] ("Scan Direction L/R")
                          }
                          frame 1 {
                            w1289 = u32 0 items=["Left to Right", "Right to Left", "Top to Bottom", "Bottom to Top"] ("Scan Direction L/R")
                          }
                        }
                        n615 = case shown="1" w1269 {
                          tunnel: [w1286 w1287] -> w1270
                          frame 0, Default {
                            w1286 = u32 2 items=["Left to Right", "Right to Left", "Top to Bottom", "Bottom to Top"] ("Scan Direction")
                          }
                          frame 1 {
                            w1287 = u32 3 items=["Left to Right", "Right to Left", "Top to Bottom", "Bottom to Top"] ("Scan Direction")
                          }
                        }
                        n616 = call "Module BL Script.vi"("Scan Direction"=w1270, "Scan Direction L/R"=w1271) -> ("In Range?"=w1273:bool, "Vertical vector"=w1277:dbl[])  [unwired: 8 in]
                        n617 = local write "Vertical vector"(w1277) -> ()
                        n618 = Select(t="Found", s=w1273, f="Failed") -> (s? t:f=w1282:string)
                        n619 = Concatenate Strings(w1279, "\r", ">", "Edge Finding", w1282) -> (w1278:string)
                      }
                      frame 6 {
                        # "HDI BL Pattern Recognition Case"
                        n620 = local read "CONTROLLER"() -> (w1291:refnum<k24>)
                        n621 = call "HDI Pat Match Full with Move BR.vi"("controller in"=w1291) -> ("In Range?"=w1290:bool)  [unwired: 11 in, 3 out]
                        n622 = Select(t="Found", s=w1290, f="Failed") -> (s? t:f=w1296:string)
                        n623 = Concatenate Strings(w1293, "\r", ">", "Pattern Matching with Move: ", w1296) -> (w1292:string)
                        n624 = local write "In Range?"(w1290) -> ()
                      }
                      frame 7 {
                        (unwired) path "C:/Users/Admin/Desktop/Main_Module_Assembly/Pattern recognition/templates/color.png" ("Template File Path")
                        # "template file"
                        # "Sensor Pattern Recognition Case"
                        n625 = local read "CONTROLLER"() -> (w1303:refnum<k24>)
                        n626 = Index Array(array=w1304, index=2) -> (element=w1300:dbl)
                        n627 = call "HDI Fiducial Full with Move.vi"("Minimum Match Score"=w1300, "controller in"=w1303) -> ("Matched?"=w1302:bool, "Score"=w1301:dbl)  [unwired: 9 in, 3 out]
                        n628 = Select(t="Found", s=w1302, f="Failed") -> (s? t:f=w1310:string)
                        n629 = Concatenate Strings(w1306, "\r", ">", "Pattern Matching with Move: ", w1310) -> (w1305:string)
                        n630 = local write "Match Score"(w1301) -> ()
                        n631 = local write "Matched?"(w1302) -> ()
                      }
                    }
                  }
                  frame 45 {
                    # "Pattern Matching for wirebonded areas"
                    n632 = Index Array(array=w1330, index #1=0 ("index"), index #2=1 ("index"), index #3=2 ("index"), index #4=3 ("index")) -> (element #1=w1322:dbl, element #2=w1321:dbl, element #3=w1320:dbl, element #4=w1314:dbl)
                    n633 = flat-sequence {
                      tunnel: w1314 -> [w1339]
                      tunnel: [w1338] -> w1316
                      tunnel: [w1337] -> w1315
                      tunnel: w1322 -> [w1379]
                      tunnel: w1321 -> [w1378]
                      tunnel: w1320 -> [w1377]
                      tunnel: [w1376] -> w1319
                      tunnel: [w1375] -> w1318
                      tunnel: [w1374] -> w1317
                      tunnel: w1316 -> [w1373]
                      tunnel: w1315 -> [w1372]
                      frame #0 {
                        # "Inputs template \nand pattern offset"
                        n634 = case shown="0, Default" w1339 {
                          tunnel: [path "C:/Documents and Settings/local-admin/Desktop/Main_Module_Assembly/Pattern recognition/wirebondFootTemp.png" ("Template File Path (Geometric Matching 1)") path "C:/Documents and Settings/local-admin/Desktop/Main_Module_Assembly/Pattern recognition/Heelrecognition.png" path "C:/Documents and Settings/local-admin/Desktop/Main_Module_Assembly/Pattern recognition/TBM HDI Whole pad RT.png" path "C:/Documents and Settings/local-admin/Desktop/Main_Module_Assembly/Pattern recognition/TBM HDI Whole pad RB.png" path "C:/Documents and Settings/local-admin/Desktop/Main_Module_Assembly/Pattern recognition/TBM HDI Whole pad BR.png" path "C:/Documents and Settings/local-admin/Desktop/Main_Module_Assembly/Pattern recognition/TBM HDI Whole pad BL.png" path "C:/Documents and Settings/local-admin/Desktop/Main_Module_Assembly/Pattern recognition/TBM HDI Whole pad LB.png" path "C:/Documents and Settings/local-admin/Desktop/Main_Module_Assembly/Pattern recognition/TBM HDI Whole pad LT.png" path "C:/Documents and Settings/local-admin/Desktop/Main_Module_Assembly/Pattern recognition/TBM HDI Whole pad TL.png" path "C:/Documents and Settings/local-admin/Desktop/Main_Module_Assembly/Pattern recognition/TBM HDI Whole pad TR.png" path "C:/Documents and Settings/local-admin/Desktop/Main_Module_Assembly/Pattern recognition/TBM TOP TR.png" path "C:/Documents and Settings/local-admin/Desktop/Main_Module_Assembly/Pattern recognition/TBM TOP BR.png" path "C:/Documents and Settings/local-admin/Desktop/Main_Module_Assembly/Pattern recognition/TBM TOP BL.png" path "C:/Documents and Settings/local-admin/Desktop/Main_Module_Assembly/Pattern recognition/TBM TOP TL.png" path "C:/Documents and Settings/local-admin/Desktop/Main_Module_Assembly/Pattern recognition/Address Bond Top.png" path "C:/Documents and Settings/local-admin/Desktop/Main_Module_Assembly/Pattern recognition/Address Bond Bottom.png"] -> w1338
                          tunnel: [cluster{"X":sgl, "Y":sgl} {"X"=0.0, "Y"=0.0} cluster{"X":sgl, "Y":sgl} {"X"=0.0, "Y"=0.0} cluster{"X":sgl, "Y":sgl} {"X"=0.0, "Y"=95.0} cluster{"X":sgl, "Y":sgl} {"X"=80.0, "Y"=0.0} cluster{"X":sgl, "Y":sgl} {"X"=0.0, "Y"=130.0} cluster{"X":sgl, "Y":sgl} {"X"=0.0, "Y"=130.0} cluster{"X":sgl, "Y":sgl} {"X"=-20.0, "Y"=0.0} cluster{"X":sgl, "Y":sgl} {"X"=-20.0, "Y"=95.0} cluster{"X":sgl, "Y":sgl} {"X"=0.0, "Y"=-75.0} cluster{"X":sgl, "Y":sgl} {"X"=15.0, "Y"=-75.0} cluster{"X":sgl, "Y":sgl} {"X"=-75.0, "Y"=-40.0} cluster{"X":sgl, "Y":sgl} {"X"=-160.0, "Y"=50.0} cluster{"X":sgl, "Y":sgl} {"X"=175.0, "Y"=0.0} cluster{"X":sgl, "Y":sgl} {"X"=160.0, "Y"=-60.0} cluster{"X":sgl, "Y":sgl} {"X"=5.0, "Y"=-180.0} cluster{"X":sgl, "Y":sgl} {"X"=0.0, "Y"=195.0}] -> w1337
                          frame 0, Default {
                          }
                          frame 1 {
                          }
                          frame 2 {
                          }
                          frame 3 {
                          }
                          frame 4 {
                          }
                          frame 5 {
                          }
                          frame 6 {
                          }
                          frame 7 {
                          }
                          frame 8 {
                          }
                          frame 9 {
                          }
                          frame 10 {
                          }
                          frame 11 {
                          }
                          frame 12 {
                          }
                          frame 13 {
                          }
                          frame 14 {
                          }
                          frame 15 {
                          }
                        }
                      }
                      frame #1 {
                        n635 = local read "CONTROLLER"() -> (w1380:refnum<k24>)
                        n636 = case shown="0, Default" w1379 {
                          tunnel: [w1387 w1394 w1403 w1411 w1417] -> w1376
                          tunnel: [w1386 w1393 w1402 w1410 w1418] -> w1374
                          tunnel: [w1385 w1395 w1401 w1409 w1419] -> w1375
                          tunnel: w1380 -> [w1382 w1391 w1400 w1406 w1416]
                          tunnel: w1378 -> [w1384 w1392 w1399 w1407 w1415]
                          tunnel: w1377 -> [w1383 w1390 w1398 w1408 w1414]
                          tunnel: w1373 -> [w1381 w1389 w1397 w1405 w1413]
                          tunnel: w1372 -> [_ w1388 w1396 w1404 w1412]
                          frame 0, Default {
                            n637 = call "WirebondPatMatch.vi"("Minimum Match Score"=w1384, "controller in"=w1382, "Template"=w1381, "Top or Bottom"=w1383) -> ("error out"=w1385:errorcluster, "Number of Matches"=w1386:i32, "Match(es) Found"=w1387:bool)  [unwired: 3 in]
                          }
                          frame 1 {
                            n638 = call "HDI Bond Match.vi"("Match Offset"=w1388, "Minimum Match Score (Pattern Matching 1)"=w1392, "controller in"=w1391, "Template"=w1389, "Numeric"=w1390) -> ("error out"=w1395:errorcluster, "Number of Matches"=w1393:i32, "Match(es) Found"=w1394:bool)  [unwired: 4 in]
                          }
                          frame 2 {
                            n639 = call "TBM HDI Wirebonds.vi"("Match Offset (Pattern Matching 1)"=w1396, "Minimum Match Score (Pattern Matching 1)"=w1399, "controller in"=w1400, "Template for Encapsulation pattern matching"=w1397, "T/B/L/R"=w1398) -> ("error out"=w1401:errorcluster, "Number of Matches (Pattern Matching 1)"=w1402:i32, "Match(es) Found"=w1403:bool)  [unwired: 4 in]
                          }
                          frame 3 {
                            n640 = call "TBM TOP.vi"("Match Offset"=w1404, "Minimum Match Score"=w1407, "controller in"=w1406, "Template"=w1405, "T/B/L/R"=w1408) -> ("error out"=w1409:errorcluster, "Number of Matches"=w1410:i32, "Match(es) Found"=w1411:bool)  [unwired: 4 in]
                          }
                          frame 4 {
                            n641 = call "Address Bond.vi"("Match Offset"=w1412, "Minimum Match Score"=w1415, "controller in"=w1416, "Template"=w1413, "T/B/L/R"=w1414) -> ("error out"=w1419:errorcluster, "Number of Matches (Pattern Matching 1)"=w1418:i32, "Match(es) Found"=w1417:bool)  [unwired: 4 in]
                          }
                        }
                      }
                    }
                    n642 = local write "error out"(w1318) -> ()
                    n643 = Select(t="Found  ", s=w1319, f="Failed  " ("t")) -> (s? t:f=w1329:string)
                    n644 = Number To Decimal String(number=w1317) -> (decimal integer string=w1328:string)  [unwired: 1 in]
                    n645 = Concatenate Strings(w1334, "\r", ">", w1329, w1328, " Matches  ") -> (w1333:string)
                  }
                  frame 46 {
                    # "Rotation correction for relative moves"
                    n646 = Index Array(array=w1456, index #1=0 ("index"), index #2=1 ("index"), index #3=2 ("index"), index #4=3 ("index")) -> (element #1=w1454:dbl, element #2=w1434:dbl, element #3=w1425:dbl, element #4=w1422:dbl)
                    n647 = local read "Stored Vectors"() -> (w1420:T1[][])
                    n648 = Index Array(array=w1420, index (col) #1=w1454, index (col) #2=w1422) -> (element #1=w1426:T1[], element #2=w1421:T1[])  [unwired: 2 in]
                    n649 = case shown="0, Default" w1425 {
                      tunnel: [w1459 w1463 w1472] -> w1443
                      tunnel: w1421 -> [_ w1468 _]
                      tunnel: w1420 -> [_ _ w1471]
                      frame 0, Default {
                        n650 = local read "Vertical vector"() -> (w1458:dbl[])
                        n651 = Array Subset(array=w1458, index=0, length=2) -> (w1457:dbl[])
                        n652 = call "2d angular offset radians.vi"("Vector 2"=dbl[] [1.0, 0.0, 0.0, 0.0], "Vector 1"=w1457) -> ("Offset Angle"=w1459:dbl)  [unwired: 9 in]
                      }
                      frame 1 {
                        n653 = Index Array(array=w1468, index=3) -> (element=w1467:T1)
                        n654 = Multiply(x=w1467, y=3.141592653589793) -> (x*y=w1465:T1)
                        n655 = Divide(x=w1465, y=180.0) -> (x/y=w1463:T1)
                      }
                      frame 2 {
                        n656 = Index Array(array=w1471, index (row)=3 ("index"), index (col)=5 ("disabled index (col)")) -> (element=w1476:T1)
                        n657 = Multiply(x=w1476, y=3.141592653589793) -> (x*y=w1474:T1)
                        n658 = Divide(x=w1474, y=180.0) -> (x/y=w1472:T1)
                      }
                    }
                    n659 = Index Array(array=w1426, index #1=0 ("index"), index #2=1 ("index")) -> (element #1=w1444:T1, element #2=w1445:T1)
                    n660 = Cosine(x=w1443) -> (cos(x)=w1451:T1)
                    n661 = Sine(x=w1443) -> (sin(x)=w1450:T1)
                    n662 = Cosine(x=w1443) -> (cos(x)=w1446:T1)
                    n663 = Sine(x=w1443) -> (sin(x)=w1447:T1)
                    n664 = Multiply(x=w1451, y=w1444) -> (x*y=w1449:T1)
                    n665 = Multiply(x=w1445, y=w1450) -> (x*y=w1448:T1)
                    n666 = Multiply(x=w1444, y=w1447) -> (x*y=w1441:T1)
                    n667 = Multiply(x=w1446, y=w1445) -> (x*y=w1442:T1)
                    n668 = Subtract(x=w1449, y=w1448) -> (x-y=w1438:T1)
                    n669 = Add(x=w1442, y=w1441) -> (x+y=w1437:T1)
                    n670 = Concatenate Strings(w1428, "\r", ">", "Rotation offset made") -> (w1427:string)
                    n671 = Build Array(w1438, w1437, 0.0 ("element"), 0.0 ("element")) -> (w1433:T1[])
                    n672 = local read "Stored Vectors"() -> (w1435:T1[][])
                    n673 = Replace Array Subset(array=w1435, new element=w1433, index (col)=w1434) -> (w1432:T1[][])  [unwired: 1 in]
                    n674 = local write "Stored Vectors"(w1432) -> ()
                  }
                  frame 47 {
                    # "Move to maintanence position"
                    n675 = local read "CONTROLLER"() -> (w1487:refnum<k24>)
                    n676 = call "Vector Mover.vi"("Absolute/Relative (F/T)"=FALSE, "Movement Vector"=dbl[] [500.0, 0.0, 0.0, 0.0], "Angular Speed"=2.0, "Vector Speed"=30.0, "controller in"=w1487) -> ()  [unwired: 1 in, 4 out]
                    n677 = Concatenate Strings(w1481, "\r", ">", "Moving to maintenance") -> (w1480:string)
                  }
                  frame 48 {
                    n678 = local read "Stored Vectors"() -> (w1506:T1[][])
                    n679 = Index Array(array=w1516) -> (element #1=w1490:dbl, element #2=w1489:dbl, element #3=w1488:dbl, element #4=w1505:dbl)  [unwired: 4 in]
                    n680 = Index Array(array=w1506, index (col)=w1490) -> (element=w1515:T1[])  [unwired: 1 in]
                    n681 = Index Array(array=w1506, index (col)=w1489) -> (element=w1509:T1[])  [unwired: 1 in]
                    n682 = Index Array(array=w1506, index (col)=w1488) -> (element=w1510:T1[])  [unwired: 1 in]
                    n683 = Number To Decimal String(number=w1490) -> (decimal integer string=w1497:string)  [unwired: 1 in]
                    n684 = Number To Decimal String(number=w1489) -> (decimal integer string=w1495:string)  [unwired: 1 in]
                    n685 = Number To Decimal String(number=w1488) -> (decimal integer string=w1493:string)  [unwired: 1 in]
                    n686 = Delete From Array(array=w1515, index=2) -> (array with subset deleted=w1513:T1[])  [unwired: 1 in, 1 out]
                    n687 = Delete From Array(array=w1509, index=2) -> (array with subset deleted=w1508:T1[])  [unwired: 1 in, 1 out]
                    n688 = Delete From Array(array=w1510, index=2) -> (array with subset deleted=w1507:T1[])  [unwired: 1 in, 1 out]
                    n689 = Concatenate Strings(w1492, "\r", ">", "finding center of circle containing tangent to points ", w1497, "," ("string"), w1495, "," ("string"), w1493) -> (w1491:string)
                    n690 = call "center of circle.vi"("point 3"=w1507, "point 2"=w1508, "point 1"=w1513) -> ("y coord"=w1503:dbl, "x coord"=w1504:dbl)  [unwired: 7 in]
                    n691 = Build Array(w1504, w1503) -> (w1502:dbl[])
                    n692 = Replace Array Subset(array=w1506, new element=w1502, index (col)=w1505) -> (w1501:T1[][])  [unwired: 1 in]
                    n693 = local write "Stored Vectors"(w1501) -> ()
                  }
                }
                n694 = Concatenate Strings(w334, "\r", "\r") -> (w340:string)
                n695 = property on="Command log" class="Str"("Value"=w340) -> ()  [unwired: 2 in, 2 out]
              }
              frame #2 {
                # "scroll to last line"
                n696 = property on="Command log" class="Str"("Text.Scroll Position"=-1) -> ()  [unwired: 2 in, 2 out]
              }
              frame #3 {
                # "increment  if in play mode and Lock is false"
                # "scroll to current line"
                # "increment command only if start/pause is true and lock is false"
                # "reset lock"
                # "forces update on play/pause button to know current\nstate"
                # "first increment commands if in play mode"
                n697 = local read "Current Command number"() -> (w1522:dbl)
                n698 = local read "Lock Increment"() -> (w1537:bool)
                n699 = local read "goto next state"() -> (w1534:bool)
                n700 = local read "Play/Pause State"() -> (w1535:bool)
                n701 = local read "step stop"() -> (w1532:bool)
                n702 = flat-sequence {
                  tunnel: w1535 -> [w1548]
                  tunnel: w1534 -> [w1547]
                  tunnel: [w1546] -> w1530
                  tunnel: [FALSE] -> w1533
                  tunnel: w1532 -> [w1544]
                  tunnel: [w1544] -> w1531
                  frame #0 {
                    # "switch mode if goto is true, pass\nstep stop into goto"
                    n703 = Not(x=w1548) -> (.not. x?=w1549:bool)
                    n704 = Select(t=w1549, s=w1547, f=w1548) -> (s? t:f=w1546:bool)
                  }
                }
                n705 = Not(x=w1537) -> (.not. x?=w1538:bool)
                n706 = And(x=w1538, y=w1535) -> (x .and. y?=w1536:bool)
                n707 = control-ref of="Command Table"() -> (w1525:refnum<vi>)
                n708 = Increment(x=w1522) -> (x+1=w1539:dbl)
                n709 = Add(x=w1522, y=1.0) -> (x+y=w1520:dbl)
                n710 = Select(t=w1539, s=w1536, f=w1522) -> (s? t:f=w1523:dbl)
                n711 = call "Color row of table.vi"("Edit Line"=w1520, "Number of Columns"=11, "Color"=u32 16448250, "Table in"=w1525) -> ()  [unwired: 7 in, 1 out]
                n712 = Select(t="||\nPause", s=w1530, f="|>\nPlay") -> (s? t:f=w1540:string)
                n713 = control-ref of="Command Table"() -> (w1524:refnum<vi>)
                n714 = local write "Current Command number"(w1523) -> ()
                n715 = property on="Start-Pause" class="Bool (strict)"("BoolText.Text"=w1540) -> ()  [unwired: 2 in, 2 out]
                n716 = local write "Lock Increment"(w1533) -> ()
                n717 = local write "goto next state"(w1531) -> ()
                n718 = local write "step stop"(w1533) -> ()
                n719 = local write "Play/Pause State"(w1530) -> ()
                n720 = Not(x=w1530) -> (.not. x?=w1543:bool)
                n721 = property on="Step Button" class="Bool (strict)"("Visible"=w1543) -> ()  [unwired: 2 in, 2 out]
                n722 = Add(x=w1523, y=1.0) -> (x+y=w1519:dbl)
                n723 = call "Color row of table.vi"("Edit Line"=w1519, "Number of Columns"=11, "Color"=u32 6618880, "Table in"=w1524) -> ()  [unwired: 7 in, 1 out]
              }
            }
          }
          frame True {
          }
        }
        n724 = local read "EXIT"() -> (w76:bool)
      }
      n725 = while {
        stop <- w32 stop-if-true
        # "get diagnostic infomation from axes"
        # "get status of touch and limit switches from axes"
        # "get position \nof axes"
        # "get faults\nfrom axes"
        n726 = local read "CONTROLLER"() -> (w23:refnum<k24>)
        n727 = call "Faults and Position data.vi"("Controller In"=w23) -> ("error out"=w22:errorcluster, "Positions"=w26:dbl[], "Faults"=w28:string[])  [unwired: 7 in, 1 out]
        n728 = local write "Faults"(w28) -> ()
        n729 = call "Touch and Limit controller.vi"("error in (no error)"=w22) -> ("error out"=w30:errorcluster, "Limit Reached"=w24:bool, "Touching"=w29:bool)  [unwired: 2 out]
        n730 = Split 1D Array(array=w26, index=4) -> (first subarray=w27:dbl[])  [unwired: 1 out]
        n731 = local write "error out"(w30) -> ()
        n732 = local write "Limit Tripped"(w24) -> ()
        n733 = local write "Touching"(w29) -> ()
        n734 = local write "Current Position"(w27) -> ()
        n735 = case shown="True" w24 {
          selector: w24 -> [_ w37]
          frame False {
          }
          frame True {
            # "if limit tripped"
            n736 = local read "CONTROLLER"() -> (w35:refnum<k24>)
            n737 = call "Abort All Movement.vi"("controller in"=w35) -> ("error out"=w36:errorcluster)  [unwired: 9 in, 1 out]
            n738 = call "Limit Reached"("Enable"=w37, "error in (no error)"=w36) -> ("Move away from surface"=w33:bool, "error out"=w34:errorcluster)  [unwired: 15 in, 1 out]
            n739 = case shown="True" w33 {
              tunnel: w35 -> [_ w39]
              tunnel: w34 -> [_ w38]
              frame False {
              }
              frame True {
                n740 = call "Vector Mover.vi"("Absolute/Relative (F/T)"=TRUE, "Movement Vector"=dbl[] [0.0, 0.0, -2.0, 0.0, 0.0], "error in (no error)"=w38, "Angular Speed"=1.0, "Vector Speed"=1.0, "controller in"=w39) -> ()  [unwired: 4 out]
              }
            }
          }
        }
        n741 = event shown="[3] \"movement abort\": Value Change" {
          selector: _ -> [_ _ _ _ _ _ _]
          dyn-events: _ -> [_ _ _ _ _ _ _]
          timeout: 100 ("t") -> [_ _ _ _ _ _ _]
          event Timeout {
            # "do nothing"
            n742 = event-data() -> ()  [unwired: 3 out]
          }
          event "Clear Log": Value Change {
            # "Clears the command log\nscreen"
            n743 = event-data() -> ()  [unwired: 6 out]
            n744 = local write "Command log"("") -> ()
            n745 = local write "Clear Log"(FALSE ("Clear Log")) -> ()
          }
          event "Start-Pause": Value Change {
            # "cause state update"
            # "Start and pause controller"
            n746 = event-data() -> ()  [unwired: 4 out]
            n747 = property on="Start-Pause" class="Bool (strict)"("Value"=FALSE) -> ()  [unwired: 2 in, 2 out]
            n748 = local write "goto next state"(TRUE) -> ()
          }
          event "movement abort": Value Change {
            # "stop all movement"
            n749 = event-data() -> ()  [unwired: 6 out]
            n750 = local read "CONTROLLER"() -> (w49:refnum<k24>)
            n751 = local write "movement abort"(FALSE ("movement abort")) -> ()
            n752 = local read "Command log"() -> (w52:string)
            n753 = call "Abort All Movement.vi"("controller in"=w49) -> ("error out"=w48:errorcluster)  [unwired: 9 in, 1 out]
            n754 = local read "Play/Pause State"() -> (w50:bool)
            n755 = Concatenate Strings(w52, "\r", ">", "Aborted all movement ") -> (w51:string)
            n756 = local write "error out"(w48) -> ()
            n757 = local write "Command log"(w51) -> ()
            n758 = case shown="True" w50 {
              frame False {
                # "do nothing in freeform"
              }
              frame True {
                # "stop if in play"
                n759 = local write "goto next state"(TRUE ("goto next state")) -> ()
              }
            }
          }
          event "Encapsulation Purge": Value Change {
            # "Controls Real Time Purge Option. Needed for encapsulation of single wires."
            n760 = event-data() -> ()  [unwired: 6 out]
            n761 = local read "Encapsulation Purge"() -> (w58:bool)
            n762 = case shown="False" w58 {
              frame False {
                n763 = local read "Command log"() -> (w63:string)
                n764 = Concatenate Strings(w63, "\r", ">" ("string"), "Encapsulation Off" ("string")) -> (w62:string)
                n765 = local write "Command log"(w62) -> ()
              }
              frame True {
                n766 = local read "Command log"() -> (w68:string)
                n767 = Concatenate Strings(w68, "\r", ">" ("string"), "Encapsulation On" ("string")) -> (w64:string)
                n768 = local write "Command log"(w64) -> ()
              }
            }
            n769 = call "Encapsulation_Control.vi"("Encapsulation  State"=w58) -> ()  [unwired: 10 in, 1 out]
            n770 = local write "Encapsulation Pressure"(w58) -> ()
          }
          event "Ack Fault": Value Change {
            # "This Acknowledges Fault and moves to a safe area on axis."
            n771 = event-data() -> ()  [unwired: 6 out]
            n772 = local read "CONTROLLER"() -> (w70:refnum<k24>)
            n773 = local read "error out"() -> (w71:errorcluster)
            n774 = call "Ack Fault.vi"("error in (no error)"=w71, "controller in"=w70) -> ("error out"=w69:errorcluster)  [unwired: 9 out]
            n775 = local write "Ack Fault"(FALSE ("Ack Fault")) -> ()
            n776 = local write "error out"(w69) -> ()
          }
          event "Step Button": Value Change {
            w73 = TRUE ("Start/Pause State")
            # "go one step through the program, then pause again"
            n777 = event-data() -> ()  [unwired: 6 out]
            n778 = local write "Step Button"(FALSE ("Step Button")) -> ()
            n779 = local write "goto next state"(w73) -> ()
            n780 = local write "step stop"(w73) -> ()
          }
        }
        n781 = local read "EXIT"() -> (w32:bool)
      }
      n782 = local read "CONTROLLER"() -> (w20:refnum<k24>)
    }
  }
  n783 = call "End Program.vi"("controller"=w1) -> ()  [unwired: 10 in, 1 out]
  n784 = local write "EXIT"(w2) -> ()
